vi "PIV_Stats.vi"() -> ()   [LabVIEW 2011]
uses:
  C:/Enflo_Software_SVN/EnFloSW/Anemometry/Anemometry Sub Vis/Controls/PIV_Spot_Data.ctl
  C:/Enflo_Software_SVN/EnFloSW/Anemometry/Anemometry Sub Vis/Controls/PIV_Spot_Cluster.ctl
  <vilib>/Utility/error.llb/DialogType.ctl
  <vilib>/Analysis/1siggen.llb/Ramp Pattern by Samples.vi
  <vilib>/Analysis/NI_AALBase.lvlib
panel:
  out "x+y":dbl[](array[numeric])
  out "size(s)":i32[](array[numeric])
  out "Position Array":dbl[][](array[numeric])
  out "Data Array":dbl[][][](array[numeric])
  out "Variable Loop":i32
  out "Collect data":i32=9857
  in  "Row number":i32=1
  out "Time Loop":i32
  out "Tmax":dbl=0.41379310344827586
  out "# bad vectors":i32[](array[numeric])
  out "# good vectors":i32[](array[numeric])
  out "Max Record Length":i32=3
  out "Numeric Control":i32=2
  out "Variable Names":string[](array[string])=["Record_Length", "CHC", "u_ms", "v_ms", "time_s", "Vel_mag_ms", "Turb_Stats_U_ms", "Turb_Stats_u2_m2s2", "Turb_Stats_u3_m3s3", "Turb_Stats_u4_m4s4", "Turb_Stats_TurbU_%", "Turb_Stats_Skew_u", "Turb_Stats_Kurt_u", "Turb_Stats_V_ms", "Turb_Stats_v2_m2s2", "Turb_Stats_v3_m3s3", "Turb_Stats_v4_m4s4", "Turb_Stats_TurbV_%", "Turb_Stats_Skew_v", "Turb_Stats_Kurt_v", "Turb_Stats_u2v2_m4s4", "Turb_Stats_uv3_m4s4", "Turb_Stats_u3v_m4s4", "Turb_Stats_uv2_m3s3", "Turb_Stats_u2v_m3s3", "Turb_Stats_uv_cc", "Turb_Stats_uv", "Turb_Stats_TKE_J", "Turb_Stats_Error_U_ms", "Turb_Stats_Error_u2_m2s2", "Turb_Stats_Error_u3_m3s3", "Turb_Stats_Error_u4_m4s4", "Turb_Stats_Error_TurbU_%", "Turb_Stats_Error_Skew_u", "Turb_Stats_Error_Kurt_u", "Turb_Stats_Error_V_ms", "Turb_Stats_Error_v2_m2s2", "Turb_Stats_Error_v3_m3s3", "Turb_Stats_Error_v4_m4s4", "Turb_Stats_Error_TurbV_%", "Turb_Stats_Error_Skew_v", "Turb_Stats_Error_Kurt_v", "Turb_Stats_Error_u2v2_m4s4", "Turb_Stats_Error_uv3_m4s4", "Turb_Stats_Error_u3v_m4s4", "Turb_Stats_Error_uv2_m3s3", "Turb_Stats_Error_u2v_m3s3", "Turb_Stats_Error_uv_cc", "Turb_Stats_Error_uv", "Turb_Stats_Error_TKE_J"]
  out "File Paths":path[][](array[path])=[[path "C:/Users/Nick/Desktop/Test/Testing/ENSI_0000.case", path "C:/Users/Nick/Desktop/Test/Testing/ENSI_0000.geo", path "C:/Users/Nick/Desktop/Test/Testing/ENSI_0000.var1", path "C:/Users/Nick/Desktop/Test/Testing/ENSI_0000.var2", path "C:/Users/Nick/Desktop/Test/Testing/ENSI_0000.var3", path "C:/Users/Nick/Desktop/Test/Testing/ENSI_0000.var4", path "C:/Users/Nick/Desktop/Test/Testing/ENSI_0000.var5", path "C:/Users/Nick/Desktop/Test/Testing/ENSI_0000.var6", path "C:/Users/Nick/Desktop/Test/Testing/ENSI_0000.var7", path "C:/Users/Nick/Desktop/Test/Testing/ENSI_0000.var8", path "C:/Users/Nick/Desktop/Test/Testing/ENSI_0000.var9", path "C:/Users/Nick/Desktop/Test/Testing/ENSI_0000.var10", path "C:/Users/Nick/Desktop/Test/Testing/ENSI_0000.var11", path "C:/Users/Nick/Desktop/Test/Testing/ENSI_0000.var12", path "C:/Users/Nick/Desktop/Test/Testing/ENSI_0000.var13", path "C:/Users/Nick/Desktop/Test/Testing/ENSI_0000.var14", path "C:/Users/Nick/Desktop/Test/Testing/ENSI_0000.var15", path "C:/Users/Nick/Desktop/Test/Testing/ENSI_0000.var16", path "C:/Users/Nick/Desktop/Test/Testing/ENSI_0000.var17", path "C:/Users/Nick/Desktop/Test/Testing/ENSI_0000.var18", path "C:/Users/Nick/Desktop/Test/Testing/ENSI_0000.var19", path "C:/Users/Nick/Desktop/Test/Testing/ENSI_0000.var20", path "C:/Users/Nick/Desktop/Test/Testing/ENSI_0000.var21", path "C:/Users/Nick/Desktop/Test/Testing/ENSI_0000.var22", path "C:/Users/Nick/Desktop/Test/Testing/ENSI_0000.var23", path "C:/Users/Nick/Desktop/Test/Testing/ENSI_0000.var24", path "C:/Users/Nick/Desktop/Test/Testing/ENSI_0000.var25", path "C:/Users/Nick/Desktop/Test/Testing/ENSI_0000.var26", path "C:/Users/Nick/Desktop/Test/Testing/ENSI_0000.var27", path "C:/Users/Nick/Desktop/Test/Testing/ENSI_0000.var28", path "C:/Users/Nick/Desktop/Test/Testing/ENSI_0000.var29", path "C:/Users/Nick/Desktop/Test/Testing/ENSI_0000.var30", path "C:/Users/Nick/Desktop/Test/Testing/ENSI_0000.var31", path "C:/Users/Nick/Desktop/Test/Testing/ENSI_0000.var32", path "C:/Users/Nick/Desktop/Test/Testing/ENSI_0000.var33", path "C:/Users/Nick/Desktop/Test/Testing/ENSI_0000.var34", path "C:/Users/Nick/Desktop/Test/Testing/ENSI_0000.var35", path "C:/Users/Nick/Desktop/Test/Testing/ENSI_0000.var36", path "C:/Users/Nick/Desktop/Test/Testing/ENSI_0000.var37", path "C:/Users/Nick/Desktop/Test/Testing/ENSI_0000.var38", path "C:/Users/Nick/Desktop/Test/Testing/ENSI_0000.var39", path "C:/Users/Nick/Desktop/Test/Testing/ENSI_0000.var40", path "C:/Users/Nick/Desktop/Test/Testing/ENSI_0000.var41", path "C:/Users/Nick/Desktop/Test/Testing/ENSI_0000.var42", path "C:/Users/Nick/Desktop/Test/Testing/ENSI_0000.var43", path "C:/Users/Nick/Desktop/Test/Testing/ENSI_0000.var44", path "C:/Users/Nick/Desktop/Test/Testing/ENSI_0000.var45", path "C:/Users/Nick/Desktop/Test/Testing/ENSI_0000.var46", path "C:/Users/Nick/Desktop/Test/Testing/ENSI_0000.var47", path "C:/Users/Nick/Desktop/Test/Testing/ENSI_0000.var48", path "C:/Users/Nick/Desktop/Test/Testing/ENSI_0000.var49", path "C:/Users/Nick/Desktop/Test/Testing/ENSI_0000.var50"], [path "C:/Users/Nick/Desktop/Test/Testing/ENSI_0001.case", path "C:/Users/Nick/Desktop/Test/Testing/ENSI_0001.geo", path "C:/Users/Nick/Desktop/Test/Testing/ENSI_0001.var1", path "C:/Users/Nick/Desktop/Test/Testing/ENSI_0001.var2", path "C:/Users/Nick/Desktop/Test/Testing/ENSI_0001.var3", path "C:/Users/Nick/Desktop/Test/Testing/ENSI_0001.var4", path "C:/Users/Nick/Desktop/Test/Testing/ENSI_0001.var5", path "C:/Users/Nick/Desktop/Test/Testing/ENSI_0001.var6", path "C:/Users/Nick/Desktop/Test/Testing/ENSI_0001.var7", path "C:/Users/Nick/Desktop/Test/Testing/ENSI_0001.var8", path "C:/Users/Nick/Desktop/Test/Testing/ENSI_0001.var9", path "C:/Users/Nick/Desktop/Test/Testing/ENSI_0001.var10", path "C:/Users/Nick/Desktop/Test/Testing/ENSI_0001.var11", path "C:/Users/Nick/Desktop/Test/Testing/ENSI_0001.var12", path "C:/Users/Nick/Desktop/Test/Testing/ENSI_0001.var13", path "C:/Users/Nick/Desktop/Test/Testing/ENSI_0001.var14", path "C:/Users/Nick/Desktop/Test/Testing/ENSI_0001.var15", path "C:/Users/Nick/Desktop/Test/Testing/ENSI_0001.var16", path "C:/Users/Nick/Desktop/Test/Testing/ENSI_0001.var17", path "C:/Users/Nick/Desktop/Test/Testing/ENSI_0001.var18", path "C:/Users/Nick/Desktop/Test/Testing/ENSI_0001.var19", path "C:/Users/Nick/Desktop/Test/Testing/ENSI_0001.var20", path "C:/Users/Nick/Desktop/Test/Testing/ENSI_0001.var21", path "C:/Users/Nick/Desktop/Test/Testing/ENSI_0001.var22", path "C:/Users/Nick/Desktop/Test/Testing/ENSI_0001.var23", path "C:/Users/Nick/Desktop/Test/Testing/ENSI_0001.var24", path "C:/Users/Nick/Desktop/Test/Testing/ENSI_0001.var25", path "C:/Users/Nick/Desktop/Test/Testing/ENSI_0001.var26", path "C:/Users/Nick/Desktop/Test/Testing/ENSI_0001.var27", path "C:/Users/Nick/Desktop/Test/Testing/ENSI_0001.var28", path "C:/Users/Nick/Desktop/Test/Testing/ENSI_0001.var29", path "C:/Users/Nick/Desktop/Test/Testing/ENSI_0001.var30", path "C:/Users/Nick/Desktop/Test/Testing/ENSI_0001.var31", path "C:/Users/Nick/Desktop/Test/Testing/ENSI_0001.var32", path "C:/Users/Nick/Desktop/Test/Testing/ENSI_0001.var33", path "C:/Users/Nick/Desktop/Test/Testing/ENSI_0001.var34", path "C:/Users/Nick/Desktop/Test/Testing/ENSI_0001.var35", path "C:/Users/Nick/Desktop/Test/Testing/ENSI_0001.var36", path "C:/Users/Nick/Desktop/Test/Testing/ENSI_0001.var37", path "C:/Users/Nick/Desktop/Test/Testing/ENSI_0001.var38", path "C:/Users/Nick/Desktop/Test/Testing/ENSI_0001.var39", path "C:/Users/Nick/Desktop/Test/Testing/ENSI_0001.var40", path "C:/Users/Nick/Desktop/Test/Testing/ENSI_0001.var41", path "C:/Users/Nick/Desktop/Test/Testing/ENSI_0001.var42", path "C:/Users/Nick/Desktop/Test/Testing/ENSI_0001.var43", path "C:/Users/Nick/Desktop/Test/Testing/ENSI_0001.var44", path "C:/Users/Nick/Desktop/Test/Testing/ENSI_0001.var45", path "C:/Users/Nick/Desktop/Test/Testing/ENSI_0001.var46", path "C:/Users/Nick/Desktop/Test/Testing/ENSI_0001.var47", path "C:/Users/Nick/Desktop/Test/Testing/ENSI_0001.var48", path "C:/Users/Nick/Desktop/Test/Testing/ENSI_0001.var49", path "C:/Users/Nick/Desktop/Test/Testing/ENSI_0001.var50"], [path "C:/Users/Nick/Desktop/Test/Testing/ENSI_0002.case", path "C:/Users/Nick/Desktop/Test/Testing/ENSI_0002.geo", path "C:/Users/Nick/Desktop/Test/Testing/ENSI_0002.var1", path "C:/Users/Nick/Desktop/Test/Testing/ENSI_0002.var2", path "C:/Users/Nick/Desktop/Test/Testing/ENSI_0002.var3", path "C:/Users/Nick/Desktop/Test/Testing/ENSI_0002.var4", path "C:/Users/Nick/Desktop/Test/Testing/ENSI_0002.var5", path "C:/Users/Nick/Desktop/Test/Testing/ENSI_0002.var6", path "C:/Users/Nick/Desktop/Test/Testing/ENSI_0002.var7", path "C:/Users/Nick/Desktop/Test/Testing/ENSI_0002.var8", path "C:/Users/Nick/Desktop/Test/Testing/ENSI_0002.var9", path "C:/Users/Nick/Desktop/Test/Testing/ENSI_0002.var10", path "C:/Users/Nick/Desktop/Test/Testing/ENSI_0002.var11", path "C:/Users/Nick/Desktop/Test/Testing/ENSI_0002.var12", path "C:/Users/Nick/Desktop/Test/Testing/ENSI_0002.var13", path "C:/Users/Nick/Desktop/Test/Testing/ENSI_0002.var14", path "C:/Users/Nick/Desktop/Test/Testing/ENSI_0002.var15", path "C:/Users/Nick/Desktop/Test/Testing/ENSI_0002.var16", path "C:/Users/Nick/Desktop/Test/Testing/ENSI_0002.var17", path "C:/Users/Nick/Desktop/Test/Testing/ENSI_0002.var18", path "C:/Users/Nick/Desktop/Test/Testing/ENSI_0002.var19", path "C:/Users/Nick/Desktop/Test/Testing/ENSI_0002.var20", path "C:/Users/Nick/Desktop/Test/Testing/ENSI_0002.var21", path "C:/Users/Nick/Desktop/Test/Testing/ENSI_0002.var22", path "C:/Users/Nick/Desktop/Test/Testing/ENSI_0002.var23", path "C:/Users/Nick/Desktop/Test/Testing/ENSI_0002.var24", path "C:/Users/Nick/Desktop/Test/Testing/ENSI_0002.var25", path "C:/Users/Nick/Desktop/Test/Testing/ENSI_0002.var26", path "C:/Users/Nick/Desktop/Test/Testing/ENSI_0002.var27", path "C:/Users/Nick/Desktop/Test/Testing/ENSI_0002.var28", path "C:/Users/Nick/Desktop/Test/Testing/ENSI_0002.var29", path "C:/Users/Nick/Desktop/Test/Testing/ENSI_0002.var30", path "C:/Users/Nick/Desktop/Test/Testing/ENSI_0002.var31", path "C:/Users/Nick/Desktop/Test/Testing/ENSI_0002.var32", path "C:/Users/Nick/Desktop/Test/Testing/ENSI_0002.var33", path "C:/Users/Nick/Desktop/Test/Testing/ENSI_0002.var34", path "C:/Users/Nick/Desktop/Test/Testing/ENSI_0002.var35", path "C:/Users/Nick/Desktop/Test/Testing/ENSI_0002.var36", path "C:/Users/Nick/Desktop/Test/Testing/ENSI_0002.var37", path "C:/Users/Nick/Desktop/Test/Testing/ENSI_0002.var38", path "C:/Users/Nick/Desktop/Test/Testing/ENSI_0002.var39", path "C:/Users/Nick/Desktop/Test/Testing/ENSI_0002.var40", path "C:/Users/Nick/Desktop/Test/Testing/ENSI_0002.var41", path "C:/Users/Nick/Desktop/Test/Testing/ENSI_0002.var42", path "C:/Users/Nick/Desktop/Test/Testing/ENSI_0002.var43", path "C:/Users/Nick/Desktop/Test/Testing/ENSI_0002.var44", path "C:/Users/Nick/Desktop/Test/Testing/ENSI_0002.var45", path "C:/Users/Nick/Desktop/Test/Testing/ENSI_0002.var46", path "C:/Users/Nick/Desktop/Test/Testing/ENSI_0002.var47", path "C:/Users/Nick/Desktop/Test/Testing/ENSI_0002.var48", path "C:/Users/Nick/Desktop/Test/Testing/ENSI_0002.var49", path "C:/Users/Nick/Desktop/Test/Testing/ENSI_0002.var50"]]
  out "ALL filepath":path=path "C:/Users/Nick/Desktop/Test/Testing/ENSI_all.case"
  in  "Invert V":bool
  in  "Invert U":bool
  in  "XYZ Translation":dbl[](array[numeric])=[0.0, 0.0, 0.0]
  in  "PIV Meas Plane":enum16{"XY", "YZ", "XZ"}(ring)=enum."XZ"
  out "time s":dbl[](array[numeric])=[0.0, 0.20689655172413793, 0.41379310344827586]
  in  "PIV Freq (Hz)":dbl=7.25
  out "File Array":path[](array[path])=[path "T:/Ensight_Data/NACA0015/NACA0015_NM_A/Test_A_Trans/New folder/Test_A000000.T076.D000.P000.H000.L.vec", path "T:/Ensight_Data/NACA0015/NACA0015_NM_A/Test_A_Trans/New folder/Test_A000001.T076.D000.P000.H000.L.vec", path "T:/Ensight_Data/NACA0015/NACA0015_NM_A/Test_A_Trans/New folder/Test_A000002.T076.D000.P000.H000.L.vec"]
  out "# total vectors":i32=9858
  in  "Case Name":string="Testing"
  in  "Data Folder":path=path "T:/Ensight_Data/NACA0015/NACA0015_NM_A/Test_A_Trans/New folder"
  in  "Output Directory":path=path "C:/Users/Nick/Desktop/Test"
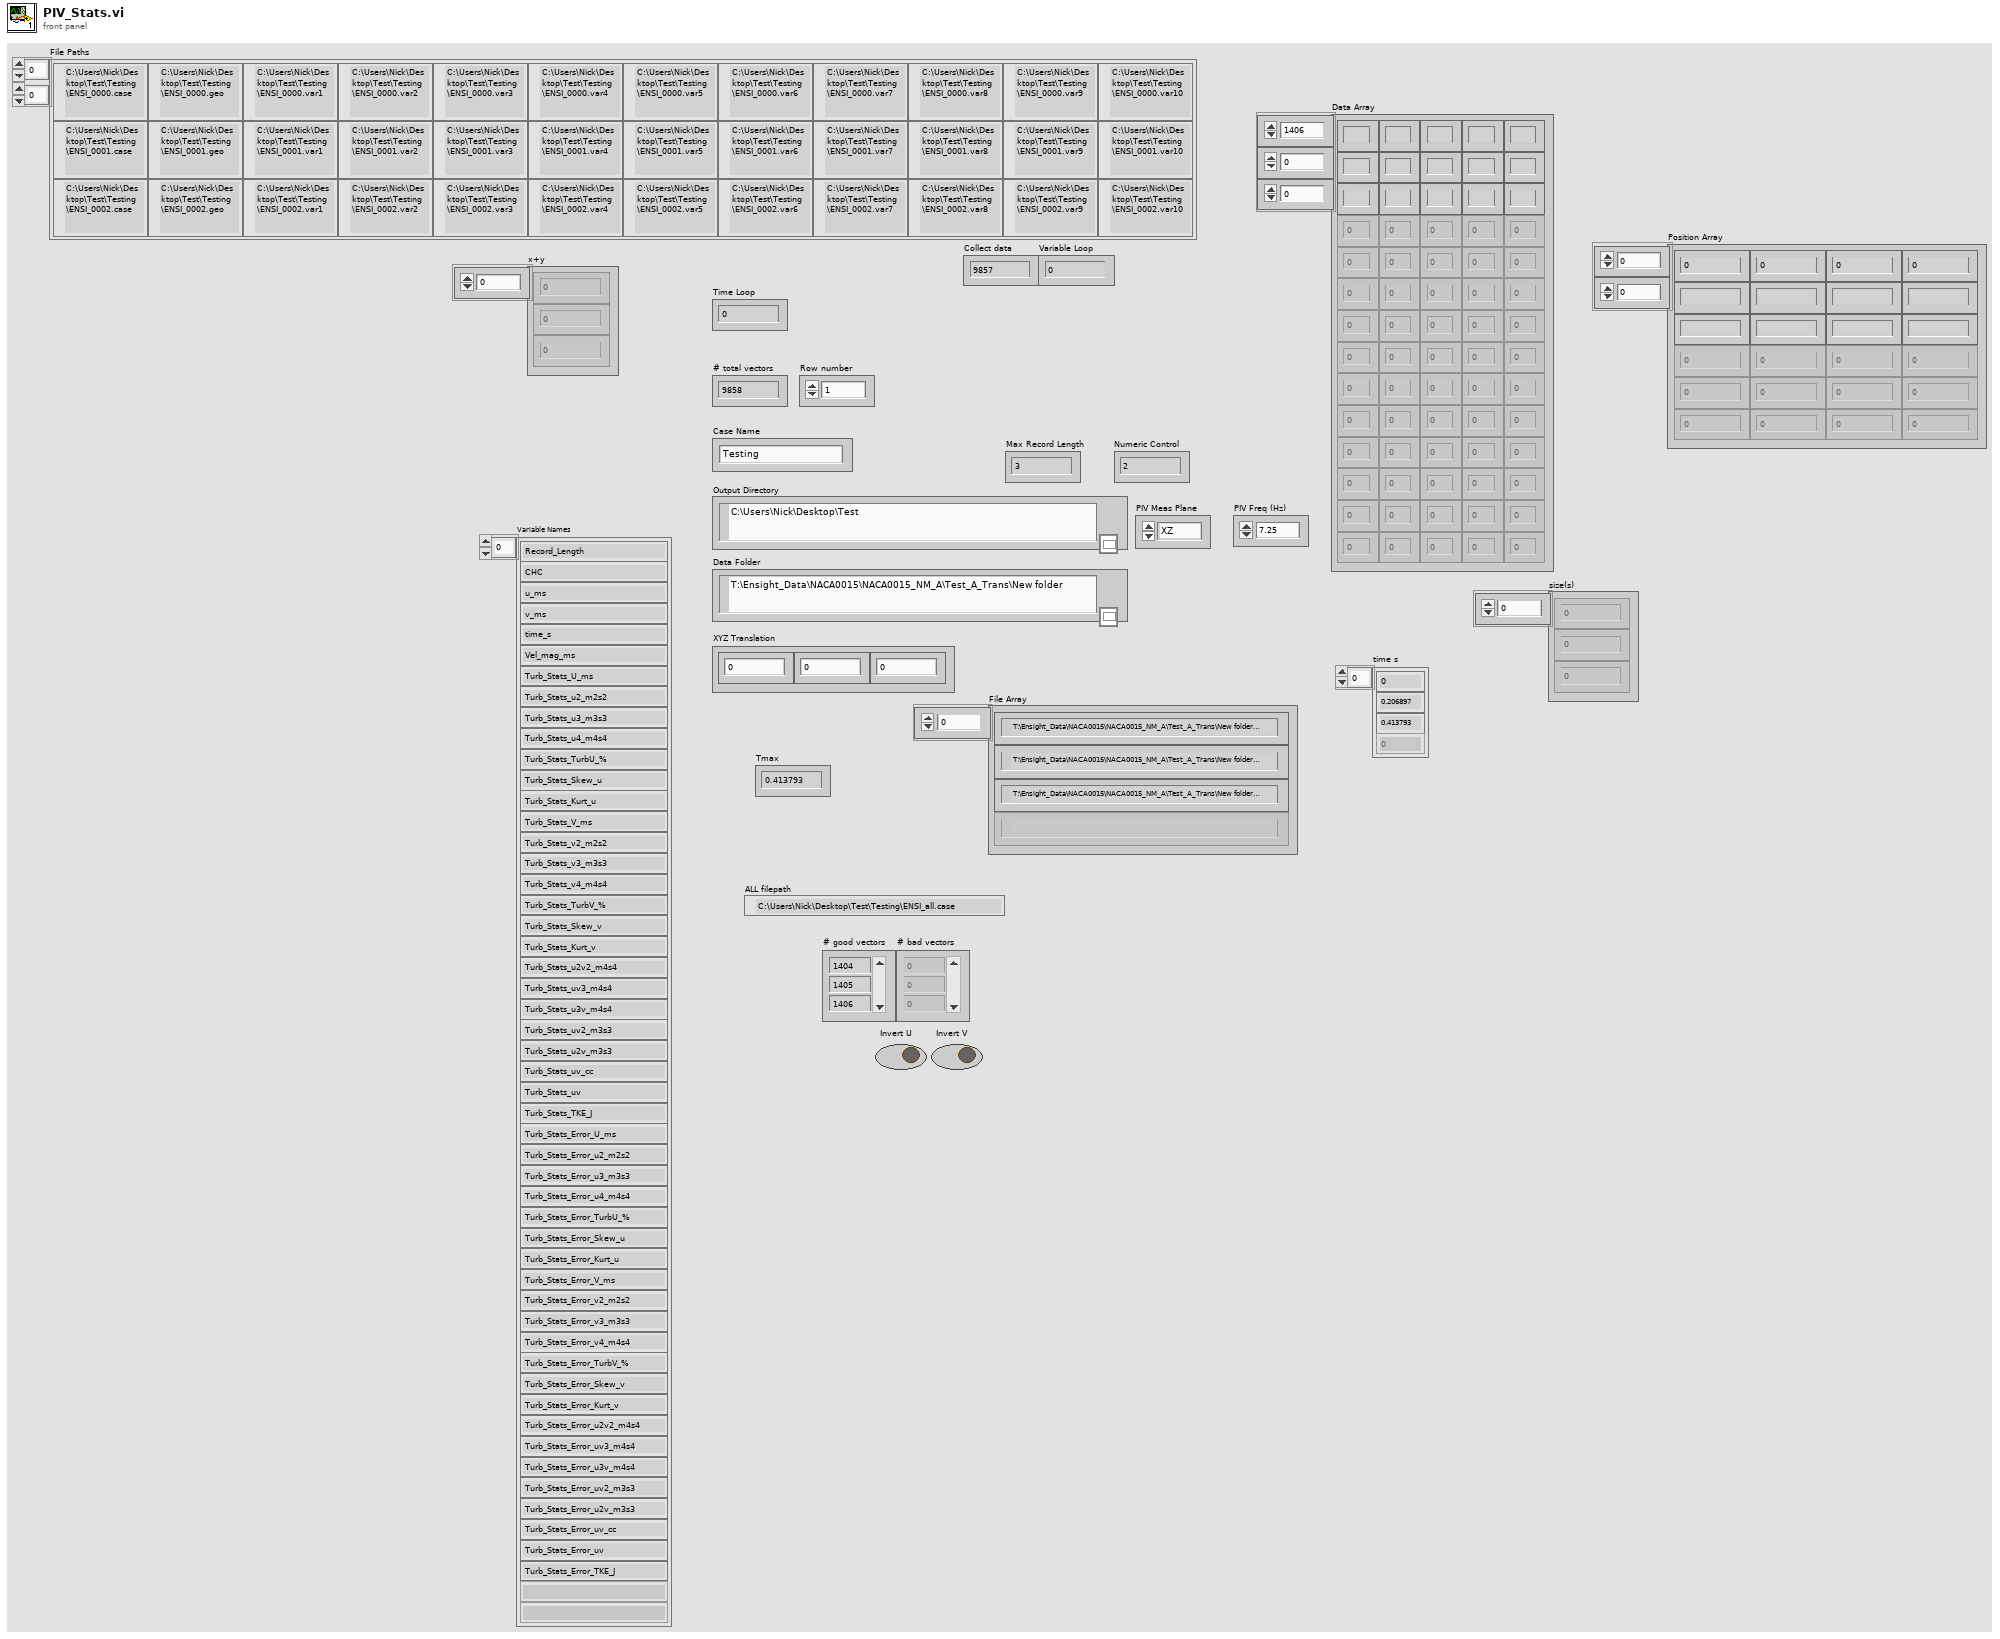
[diagram p1: front panel]
types:
  T1 = typedef "PIV_Spot_Data.ctl" = T2[]
  T2 = typedef "PIV_Spot_Cluster.ctl" = cluster{"Record Length":dbl, "CHC":dbl[], "u m/s":dbl[], "v m/s":dbl[], "time s":dbl[], "Vel mag m/s":dbl[], "XYZ Position":dbl[], " Turb Stats":cluster{"U m/s":dbl, "u2 m2/s2":dbl, "u3 m3/s3":dbl, "u4 m4/s4":dbl, "TurbU %":dbl, "Skew_u":dbl, "Kurt_u":dbl, "V m/s":dbl, "v2 m2/s2":dbl, "v3 m3/s3":dbl, "v4 m4/s4":dbl, "TurbV %":dbl, "Skew_v":dbl, "Kurt_v":dbl, "u2v2 m4/s4":dbl, "uv3 m4/s4":dbl, "u3v m4/s4":dbl, "uv2 m3/s3":dbl, "u2v m3/s3":dbl, "uv_cc":dbl, "uv":dbl, "TKE J":dbl}[], "Turb Stats Error":cluster{"U m/s":dbl, "u2 m2/s2":dbl, "u3 m3/s3":dbl, "u4 m4/s4":dbl, "TurbU %":dbl, "Skew_u":dbl, "Kurt_u":dbl, "V m/s":dbl, "v2 m2/s2":dbl, "v3 m3/s3":dbl, "v4 m4/s4":dbl, "TurbV %":dbl, "Skew_v":dbl, "Kurt_v":dbl, "u2v2 m4/s4":dbl, "uv3 m4/s4":dbl, "u3v m4/s4":dbl, "uv2 m3/s3":dbl, "u2v m3/s3":dbl, "uv_cc":dbl, "uv":dbl, "TKE J":dbl}[]}
  T3 = cluster{"U m/s":dbl, "u2 m2/s2":dbl, "u3 m3/s3":dbl, "u4 m4/s4":dbl, "TurbU %":dbl, "Skew_u":dbl, "Kurt_u":dbl, "V m/s":dbl, "v2 m2/s2":dbl, "v3 m3/s3":dbl, "v4 m4/s4":dbl, "TurbV %":dbl, "Skew_v":dbl, "Kurt_v":dbl, "u2v2 m4/s4":dbl, "uv3 m4/s4":dbl, "u3v m4/s4":dbl, "uv2 m3/s3":dbl, "u2v m3/s3":dbl, "uv_cc":dbl, "uv":dbl, "TKE J":dbl}
  T4 = cluster{"U m/s":dbl, "u2 m2/s2":dbl, "u3 m3/s3":dbl, "u4 m4/s4":dbl, "TurbU %":dbl, "Skew_u":dbl, "Kurt_u":dbl, "V m/s":dbl, "v2 m2/s2":dbl, "v3 m3/s3":dbl, "v4 m4/s4":dbl, "TurbV %":dbl, "Skew_v":dbl, "Kurt_v":dbl, "u2v2 m4/s4":dbl, "uv3 m4/s4":dbl, "u3v m4/s4":dbl, "uv2 m3/s3":dbl, "u2v m3/s3":dbl, "uv_cc":dbl, "uv":dbl, "TKE J":dbl}[]
  T5 = typedef "DialogType.ctl" = u16
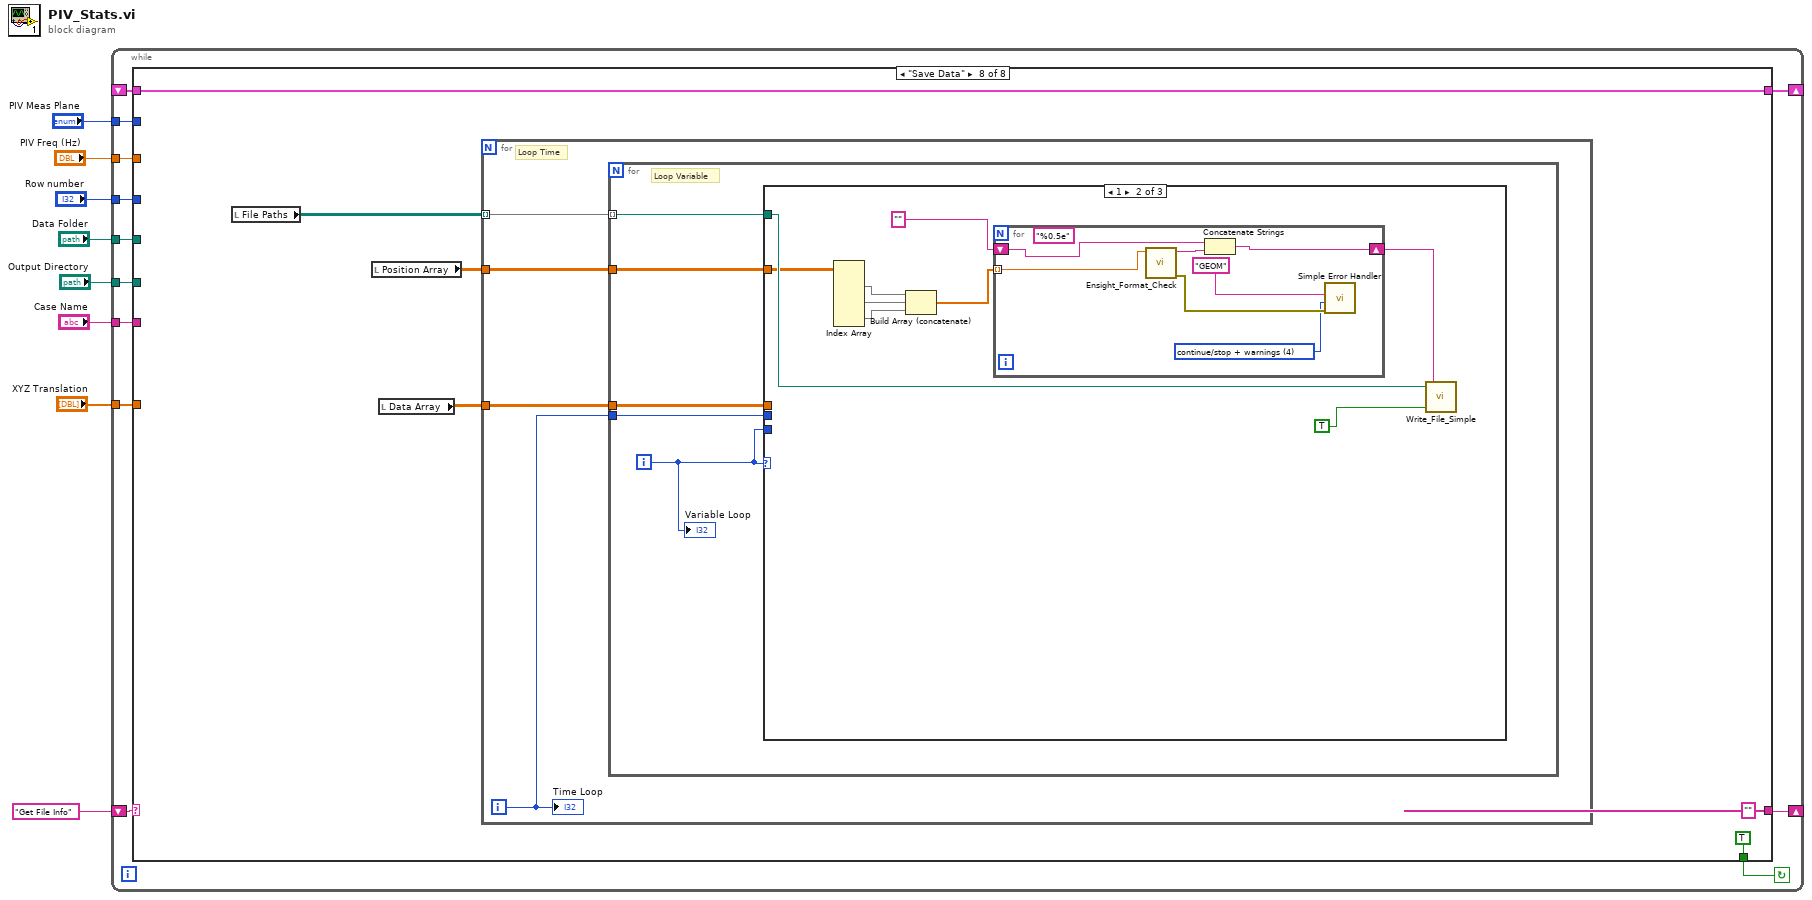
[diagram p0: block diagram]
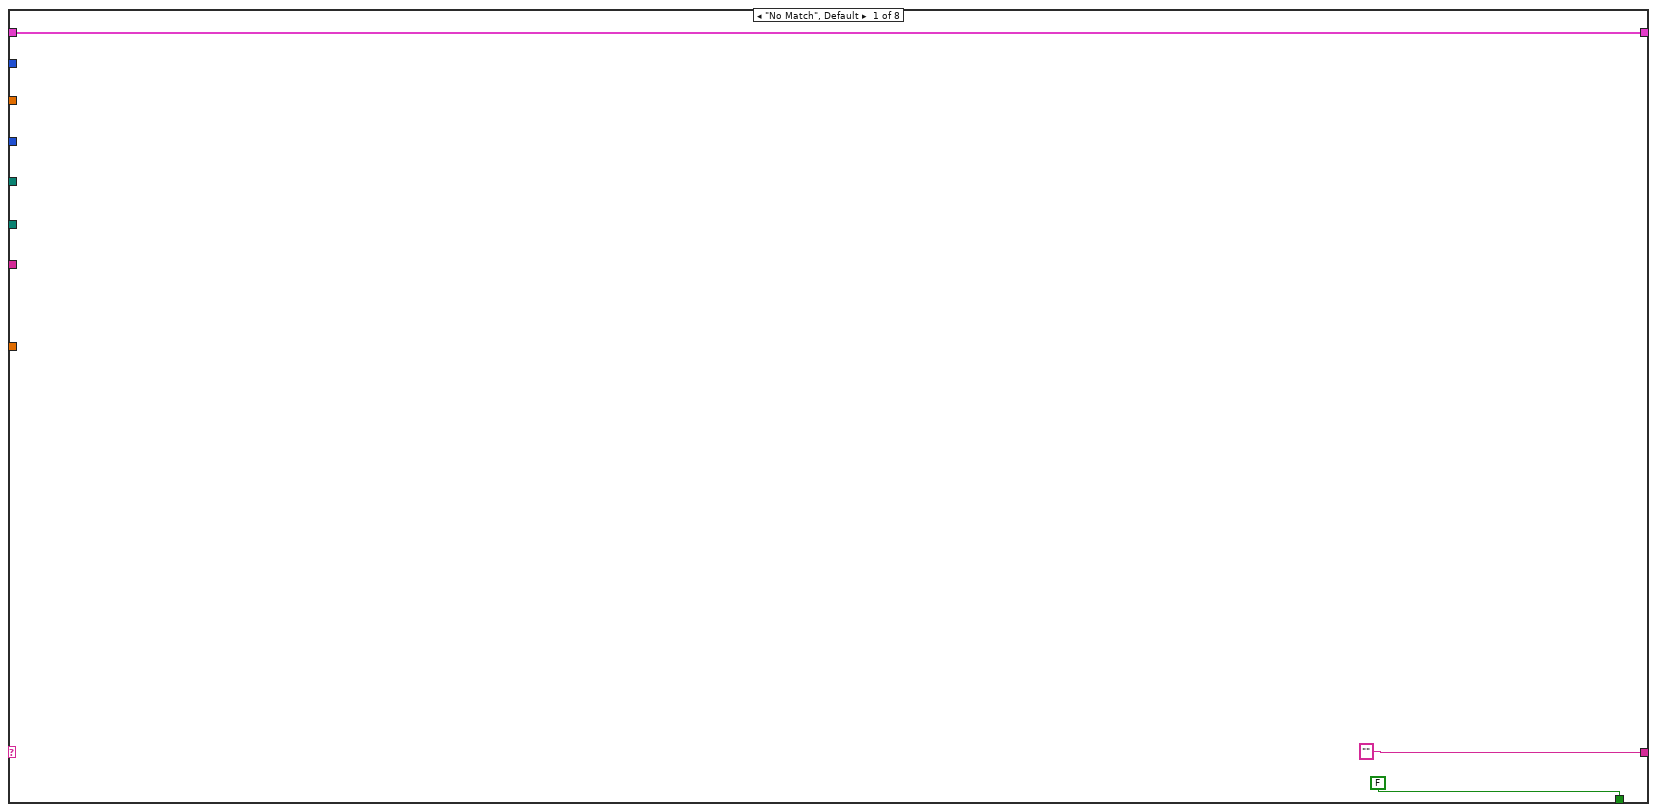
[diagram p2: hidden frame]
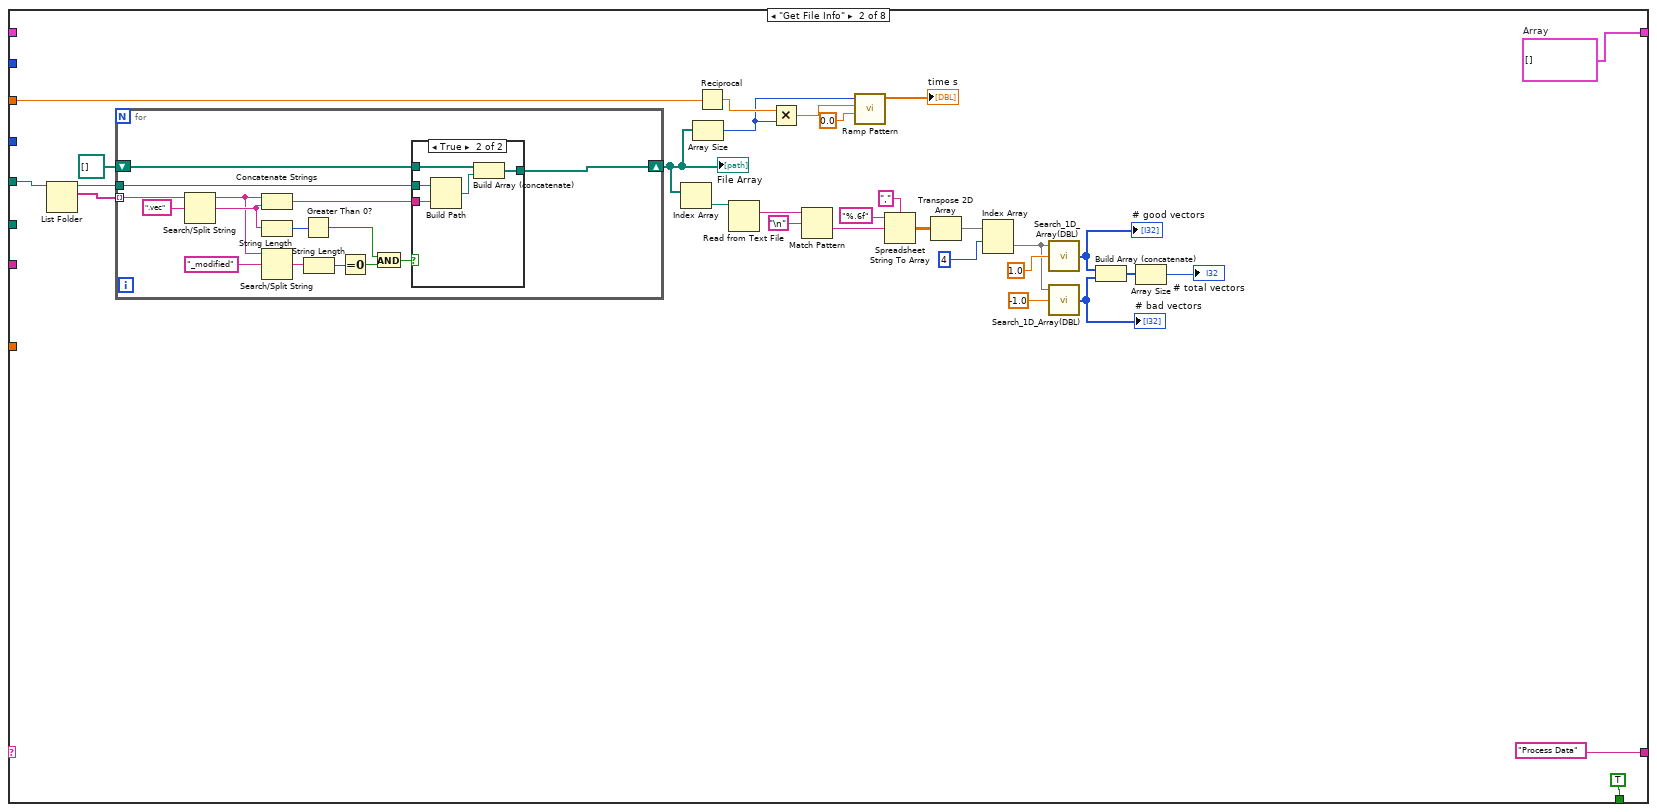
[diagram p3: hidden frame]
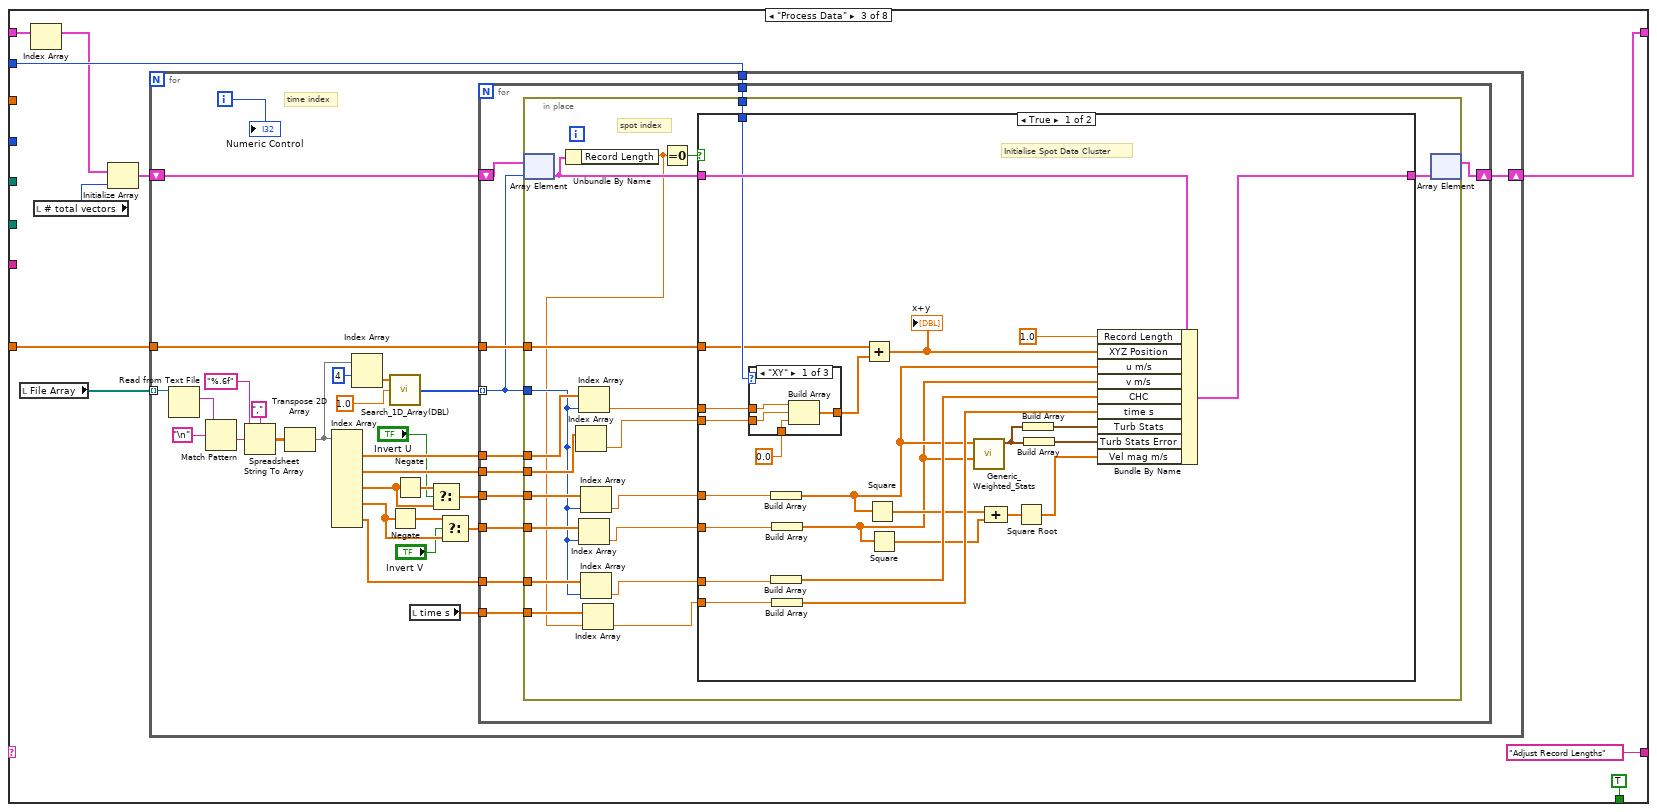
[diagram p5: hidden frame]
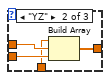
[diagram p6: hidden frame]
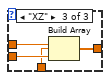
[diagram p7: hidden frame]
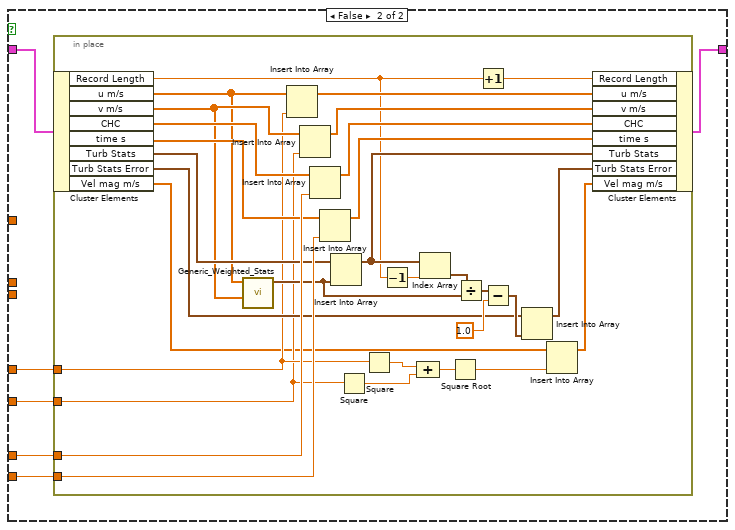
[diagram p8: hidden frame]
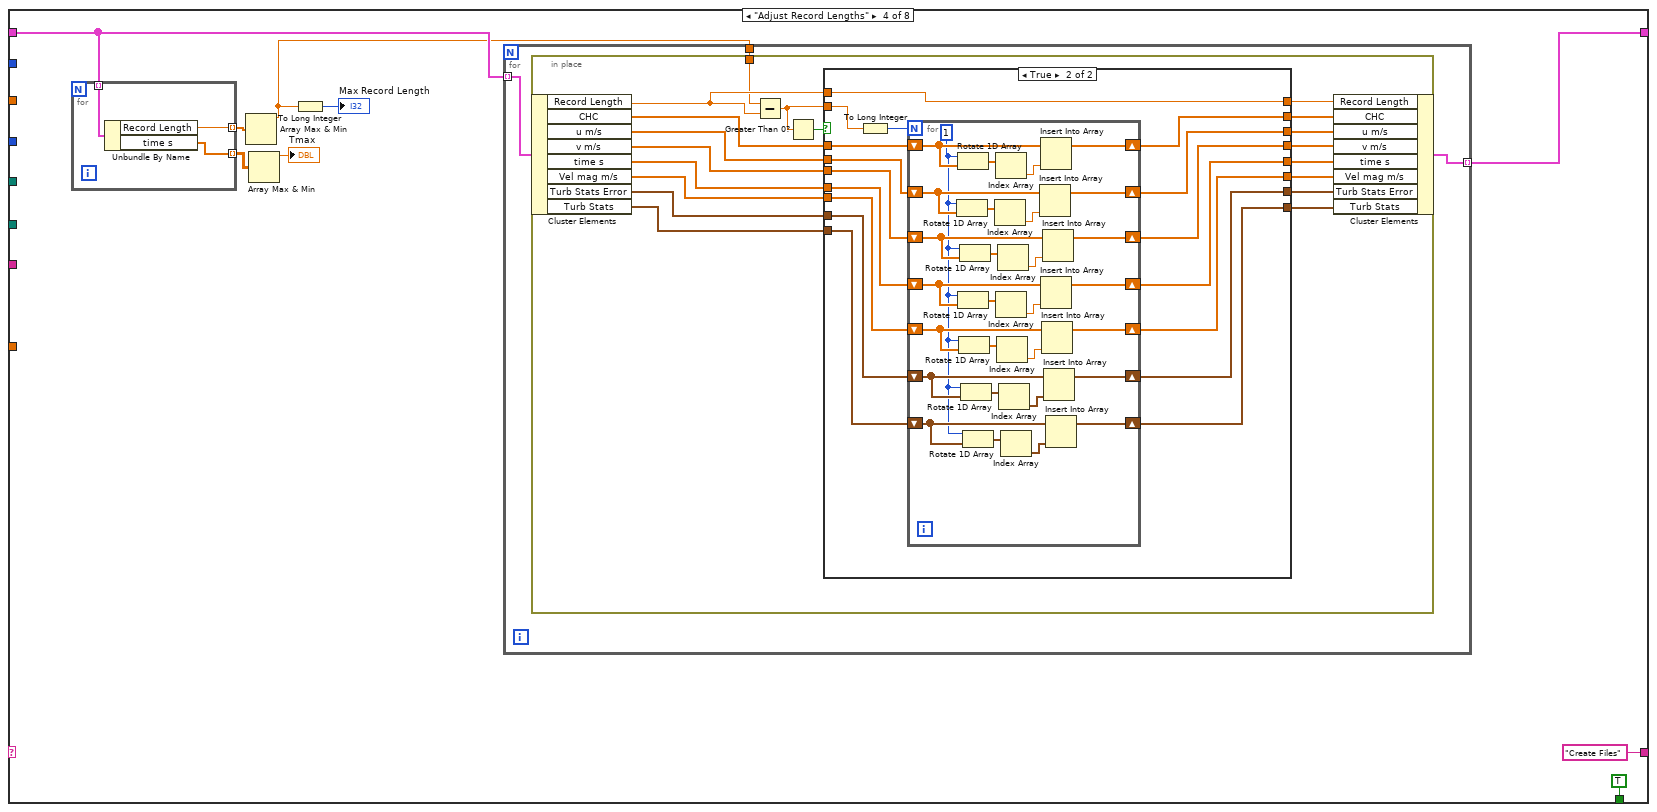
[diagram p9: hidden frame]
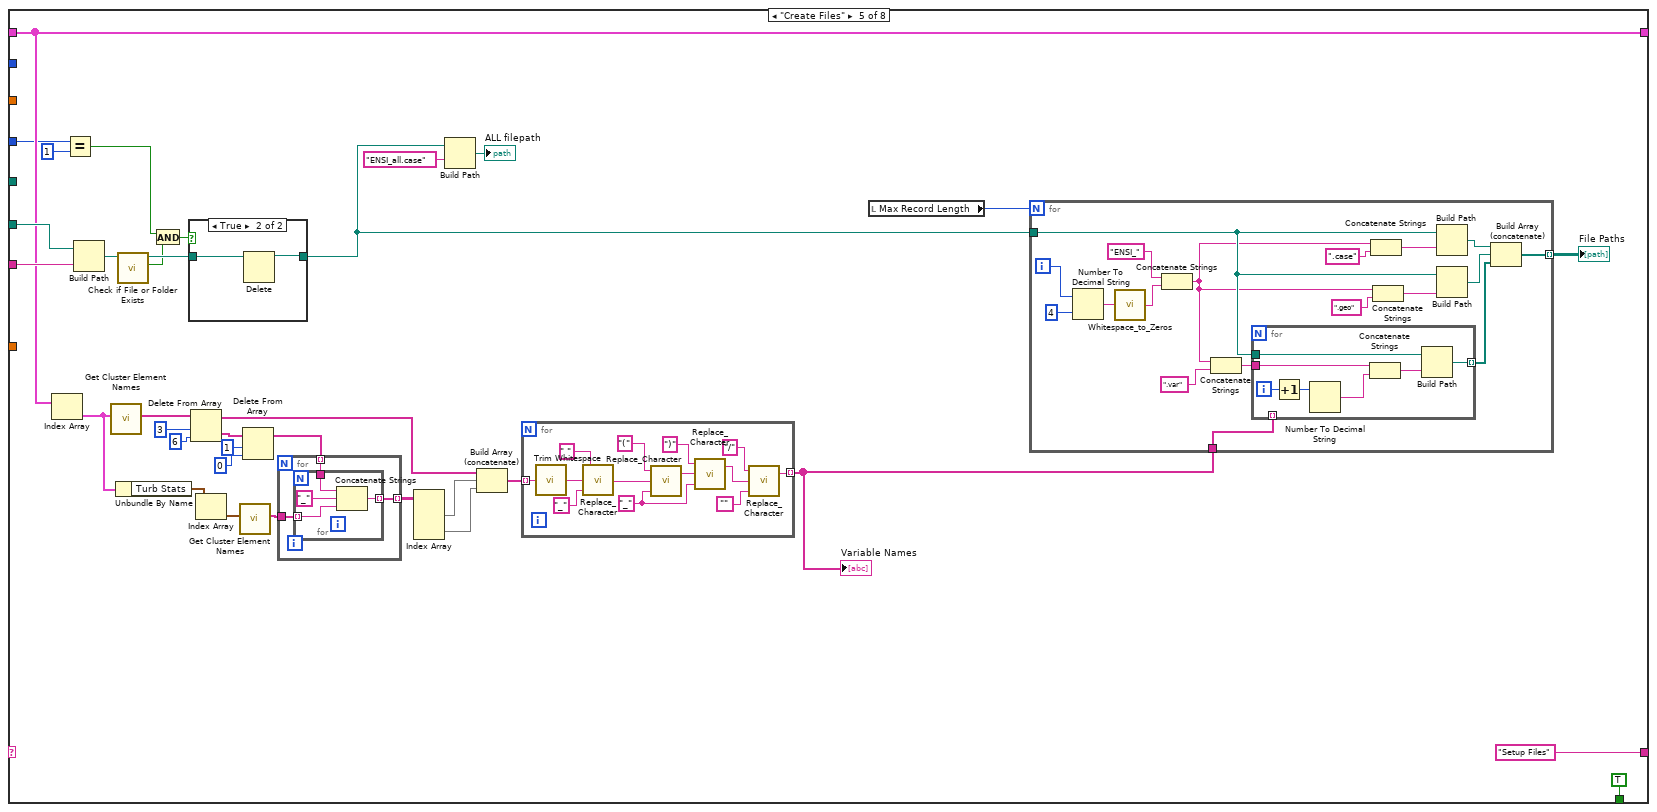
[diagram p11: hidden frame]
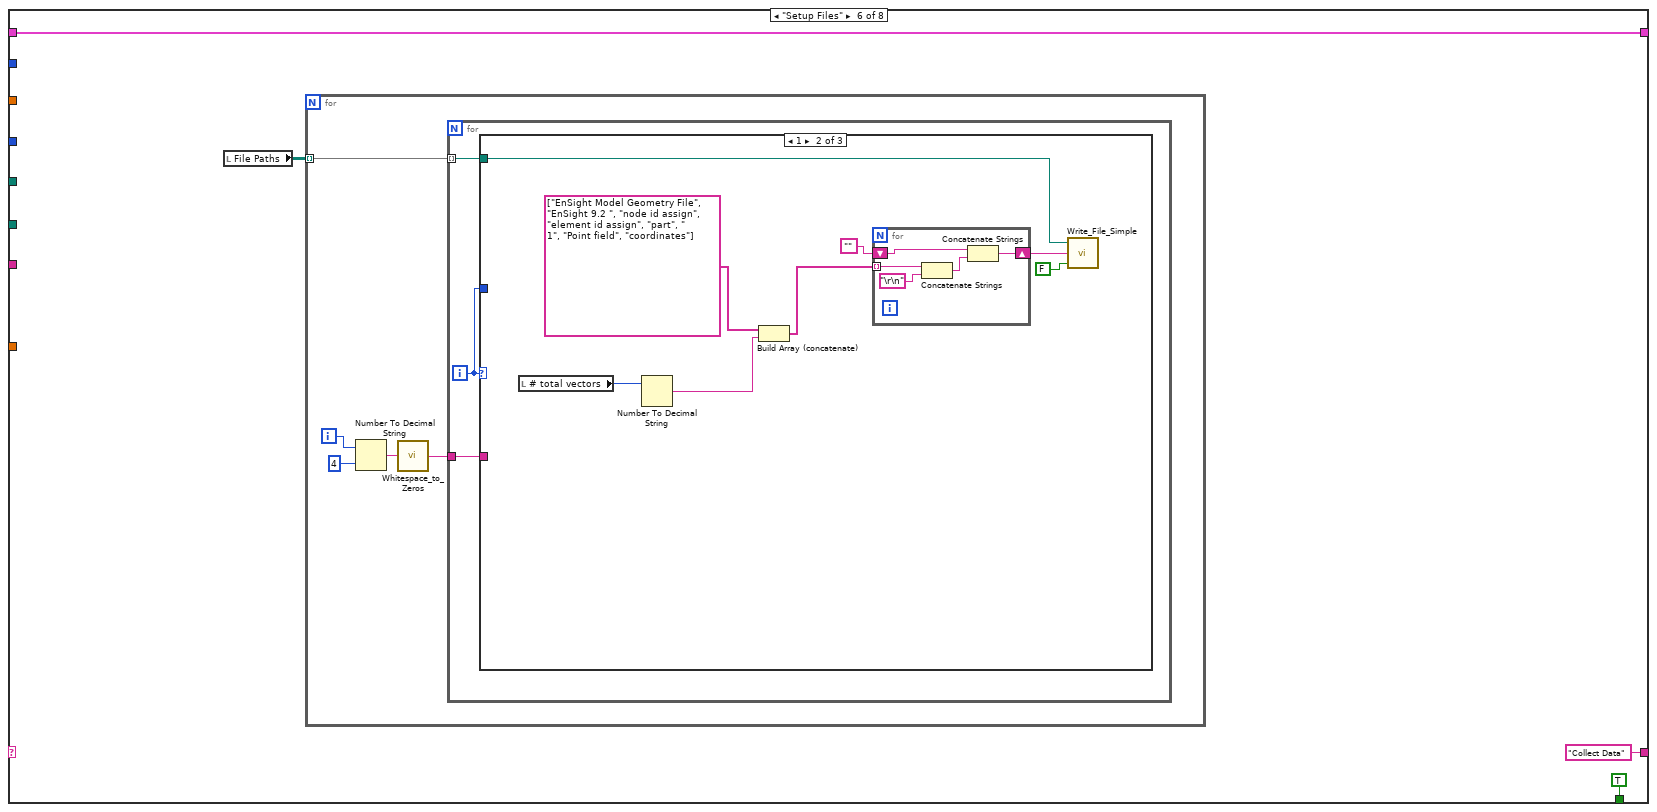
[diagram p13: hidden frame]
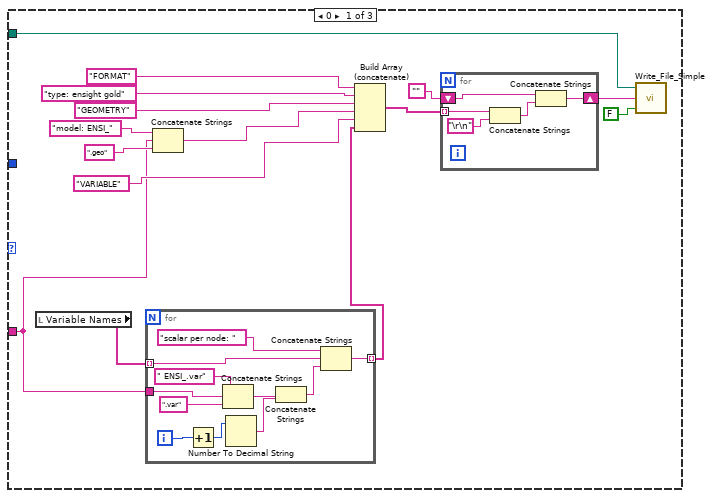
[diagram p14: hidden frame]
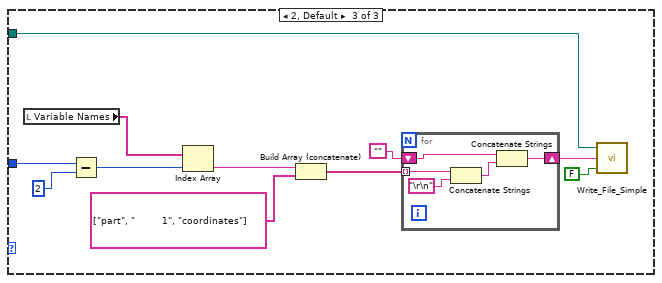
[diagram p15: hidden frame]
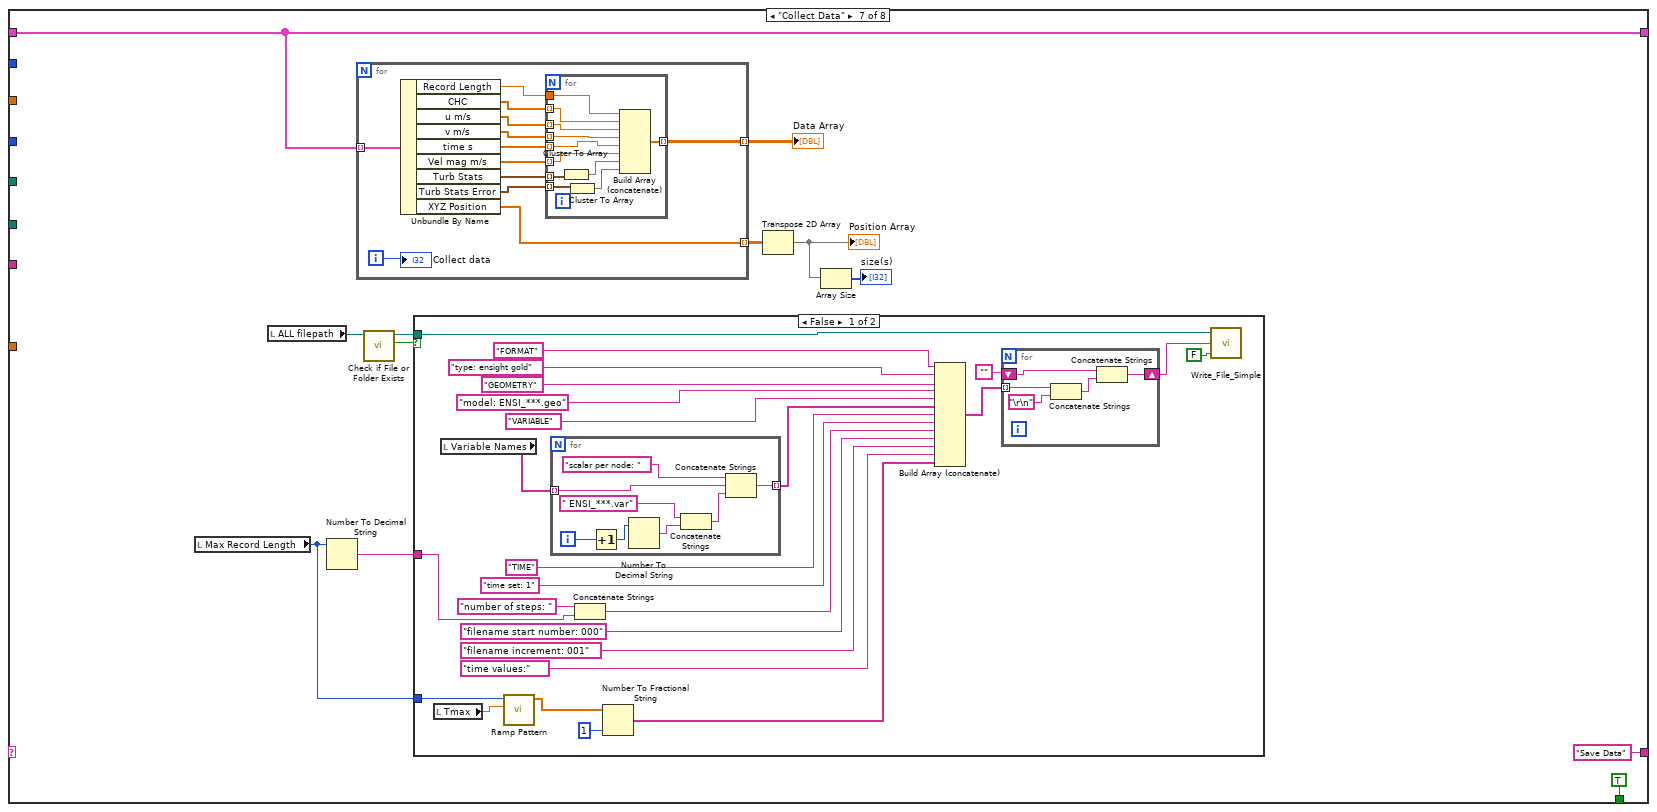
[diagram p16: hidden frame]
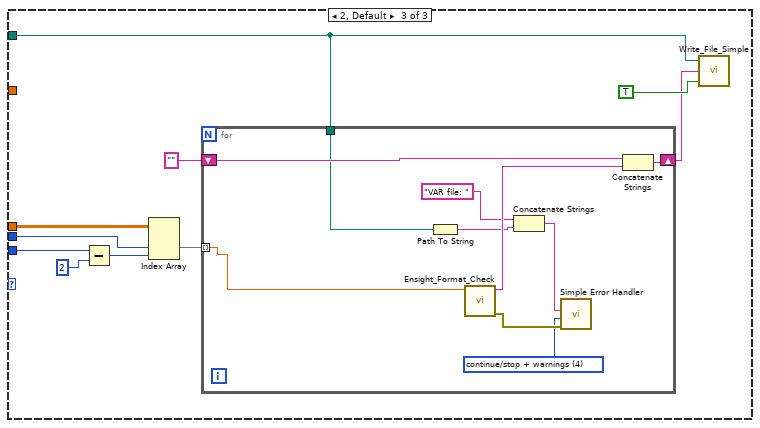
[diagram p19: hidden frame]
diagram:
  n1 = while {
    shift-right: [w19] -> _
    shift-left: "Get File Info" -> [w20]
    tunnel: "Data Folder" -> [w18]
    tunnel: "Output Directory" -> [w16]
    tunnel: "Case Name" -> [w15]
    tunnel: "PIV Freq (Hz)" -> [w14]
    tunnel: "PIV Meas Plane" -> [w13]
    tunnel: "XYZ Translation" -> [w12]
    shift-right: [w11] -> _
    shift-left: _ -> [w10]
    tunnel: "Row number" -> [w9]
    stop <- w17 continue-if-true
    n2 = case shown="\"Save Data\"" w20 {
      tunnel: ["" "Process Data" "Adjust Record Lengths" "Create Files" "Setup Files" ("t") "Collect Data" ("t") "Save Data" ("t") "" ("t")] -> w19
      tunnel: w18 -> [_ w48 _ _ _ _ _ _]
      tunnel: [FALSE TRUE TRUE TRUE TRUE TRUE TRUE TRUE] -> w17
      tunnel: w16 -> [_ _ _ _ w334 _ _ _]
      tunnel: w15 -> [_ _ _ _ w335 _ _ _]
      tunnel: w14 -> [_ w41 _ _ _ _ _ _]
      tunnel: w13 -> [_ _ w80 _ _ _ _ _]
      tunnel: w12 -> [_ _ w79 _ _ _ _ _]
      tunnel: [w21 w25 w77 w223 w318 w387 w463 w535] -> w11
      tunnel: w10 -> [w21 _ w76 w222 w318 w387 w463 w535]
      tunnel: w9 -> [_ _ _ _ w313 _ _ _]
      frame "No Match", Default {
      }
      frame "Get File Info" {
        w25 = T1 []  # Array
        n3 = List Folder(path=w48) -> (path out=w50:path, filenames=w51:string[])  [unwired: 3 in, 2 out]
        n4 = for {
          tunnel: w51 -> [w68] mode=indexing
          shift-right: [w61] -> w33
          shift-left: path[] [] -> [w63]
          tunnel: w50 -> [w62]
          n5 = Search/Split String(string=w68, search string/char (-)=".vec") -> (substring before match=w59:string, match + rest of string=w65:string)  [unwired: 1 in, 1 out]
          n6 = Concatenate Strings(w59, w65) -> (w64:string)
          n7 = String Length(string=w65) -> (length=w66:i32)
          n8 = Search/Split String(string=w59, search string/char (-)="_modified") -> (match + rest of string=w57:string)  [unwired: 1 in, 2 out]
          n9 = Greater Than 0?(x=w66) -> (x > 0?=w60:bool)
          n10 = String Length(string=w57) -> (length=w56:i32)
          n11 = Equal To 0?(x=w56) -> (x = 0?=w55:bool)
          n12 = And(x=w60, y=w55) -> (x .and. y?=w54:bool)
          n13 = case shown="True" w54 {
            tunnel: w64 -> [_ w74]
            tunnel: w63 -> [w69 w70]
            tunnel: w62 -> [_ w73]
            tunnel: [w69 w71] -> w61
            frame False {
            }
            frame True {
              n14 = Build Path(base path=w73, name or relative path=w74) -> (appended path=w72:path)
              n15 = Build Array (concatenate)(w70, w72) -> (w71:path[])
            }
          }
        }
        "File Array" <- w33
        n16 = Index Array(array=w33) -> (element=w42:path)  [unwired: 1 in]
        n17 = Array Size(array=w33) -> (size(s)=w30:i32)
        n18 = Reciprocal(x=w41) -> (1/x=w39:dbl)
        n19 = Read from Text File(file (use dialog)=w42) -> (text=w47:string)  [unwired: 3 in, 3 out]
        n20 = Multiply(x=w39, y=w30) -> (x*y=w40:dbl)
        n21 = Match Pattern(string=w47, regular expression="\n") -> (after substring=w43:string)  [unwired: 1 in, 3 out]
        n22 = call-poly <vilib>:"Ramp Pattern.vi"("start"=0.0, "end"=w40, "samples"=w30) -> ("Ramp Pattern"=→"time s":dbl[])  [unwired: 7 in, 1 out]
        n23 = Spreadsheet String To Array(delimiter (Tab)=",", format string="%.6f", spreadsheet string=w43) -> (array=w34:dbl[][])  [unwired: 1 in]
        n24 = Transpose 2D Array(2D array=w34) -> (transposed array=w36:dbl[][])
        n25 = Index Array(array=w36, index (row)=4) -> (element=w29:dbl[])  [unwired: 1 in]
        n26 = call "Search_1D_Array(DBL).vi"("Array"=w29, "Element Data"=1.0) -> ("Indicies of Elements"=w27:i32[])  [unwired: 7 in]
        "# good vectors" <- w27
        n27 = call "Search_1D_Array(DBL).vi"("Array"=w29, "Element Data"=-1.0) -> ("Indicies of Elements"=w24:i32[])  [unwired: 7 in]
        "# bad vectors" <- w24
        n28 = Build Array (concatenate)(w27, w24) -> (w26:i32[])
        n29 = Array Size(array=w26) -> (size(s)=→"# total vectors":i32)
      }
      frame "Process Data" {
        n30 = local read "File Array"() -> (w81:path[])
        n31 = Index Array(array=w76) -> (element=w75:T2)  [unwired: 1 in]
        n32 = local read "# total vectors"() -> (w78:i32)
        n33 = Initialize Array(w75, w78) -> (w82:T2[])
        n34 = for {
          tunnel: w81 -> [w113] mode=indexing
          shift-right: [w89] -> w77
          shift-left: w82 -> [w106]
          tunnel: w80 -> [w101]
          tunnel: w79 -> [w100]
          i -> [w86]
          # "time index"
          n35 = Read from Text File(file (use dialog)=w113) -> (text=w107:string)  [unwired: 3 in, 3 out]
          n36 = Match Pattern(string=w107, regular expression="\n") -> (after substring=w111:string)  [unwired: 1 in, 3 out]
          n37 = Spreadsheet String To Array(delimiter (Tab)=",", format string="%.6f", spreadsheet string=w111) -> (array=w112:dbl[][])  [unwired: 1 in]
          n38 = Transpose 2D Array(2D array=w112) -> (transposed array=w99:dbl[][])
          n39 = Index Array(array=w99) -> (element #1=w103:dbl[], element #2=w102:dbl[], element #3=w98:dbl[], element #4=w95:dbl[], element #5=w92:dbl[])  [unwired: 10 in]
          n40 = Index Array(array=w99, index (row)=4) -> (element=w88:dbl[])  [unwired: 1 in]
          n41 = call "Search_1D_Array(DBL).vi"("Array"=w88, "Element Data"=1.0) -> ("Indicies of Elements"=w85:i32[])  [unwired: 7 in]
          n42 = Negate(x=w95) -> (-x=w96:dbl[])
          n43 = Negate(x=w98) -> (-x=w97:dbl[])
          n44 = local read "time s"() -> (w104:dbl[])
          n45 = Select(t=w97, s="Invert U", f=w98) -> (s? t:f=w91:dbl[])
          n46 = Select(t=w96, s="Invert V", f=w95) -> (s? t:f=w90:dbl[])
          n47 = for {
            tunnel: w104 -> [w117]
            tunnel: w103 -> [w124]
            tunnel: w102 -> [w123]
            tunnel: w101 -> [w122]
            tunnel: w100 -> [w121]
            tunnel: w92 -> [w118]
            tunnel: w91 -> [w120]
            tunnel: w90 -> [w119]
            tunnel: w85 -> [w114] mode=indexing
            shift-right: [w115] -> w89
            shift-left: w106 -> [w116]
            n48 = in-place {
              in-place-border: w124 -> [w143]
              in-place-border: w123 -> [w142]
              in-place-border: w122 -> [w141]
              in-place-border: w121 -> [w140]
              in-place-border: w120 -> [w139]
              in-place-border: w119 -> [w138]
              in-place-border: w118 -> [w137]
              in-place-border: w117 -> [w136]
              in-place-border: w114 -> [w126]
              # "spot index"
              n49 = in-place-array #1(w116, w114) -> (w128:T2)
              n50 = Unbundle By Name(w128) -> ("Record Length"=w125:dbl)
              n51 = Index Array(array=w142, index=w126) -> (element=w134:dbl)
              n52 = Index Array(array=w143, index=w126) -> (element=w135:dbl)
              n53 = Index Array(array=w138, index=w126) -> (element=w132:dbl)
              n54 = Index Array(array=w139, index=w126) -> (element=w133:dbl)
              n55 = Index Array(array=w137, index=w126) -> (element=w131:dbl)
              n56 = Index Array(array=w136, index=w125) -> (element=w130:dbl)
              n57 = Equal To 0?(x=w125) -> (x = 0?=w129:bool)
              n58 = case shown="True" w129 {
                tunnel: [w167 w186] -> w127
                tunnel: w132 -> [w155 w183]
                tunnel: w128 -> [w168 w185]
                tunnel: w135 -> [w164 _]
                tunnel: w134 -> [w163 _]
                tunnel: w141 -> [w165 _]
                tunnel: w140 -> [w161 _]
                tunnel: w133 -> [w158 w184]
                tunnel: w131 -> [w157 w182]
                tunnel: w130 -> [w154 w181]
                frame True {
                  # "Initialise Spot Data Cluster"
                  n59 = case shown="\"XY\"" w165 {
                    tunnel: w164 -> [w170 w176 w180]
                    tunnel: w163 -> [w171 w175 w179]
                    tunnel: 0.0 ("element") -> [w172 w174 w178]
                    tunnel: [w169 w173 w177] -> w162
                    frame "XY" {
                      n60 = Build Array(w170, w171, w172) -> (w169:dbl[])
                    }
                    frame "YZ" {
                      n61 = Build Array(w174, w176, w175) -> (w173:dbl[])
                    }
                    frame "XZ" {
                      n62 = Build Array(w180, w178, w179) -> (w177:dbl[])
                    }
                  }
                  n63 = Build Array(w158) -> (w149:dbl[])
                  n64 = Build Array(w157) -> (w156:dbl[])
                  n65 = Build Array(w155) -> (w147:dbl[])
                  n66 = Build Array(w154) -> (w153:dbl[])
                  n67 = Add(x=w161, y=w162) -> (x+y=w160:dbl[])
                  "x+y" <- w160
                  n68 = Square(x=w149) -> (x^2=w148:dbl[])
                  n69 = Square(x=w147) -> (x^2=w146:dbl[])
                  n70 = call "Generic_Weighted_Stats.vi"("v"=w147, "u"=w149) -> ("Turbulence Statistics"=w151:T3)  [unwired: 9 in]
                  n71 = Compound Arithmetic op=ADD(w148, w146) -> (w145:dbl[])
                  n72 = Square Root(x=w145) -> (sqrt(x)=w144:dbl[])
                  n73 = Build Array(w151) -> (w152:T4)
                  n74 = Build Array(w151) -> (w150:T4)
                  n75 = Bundle By Name(cluster=w168, "Record Length"=1.0, "XYZ Position"=w160, "u m/s"=w149, "v m/s"=w147, "CHC"=w156, "time s"=w153, "Turb Stats"=w152, "Turb Stats Error"=w150, "Vel mag m/s"=w144) -> (w167:T2)
                }
                frame False {
                  n76 = in-place {
                    in-place-border: w184 -> [w193]
                    in-place-border: w183 -> [w192]
                    in-place-border: w182 -> [w213]
                    in-place-border: w181 -> [w211]
                    n77 = in-place-cluster #2(w185) -> ("Record Length"=w204:dbl, "u m/s"=w206:dbl[], "v m/s"=w207:dbl[], "CHC"=w214:dbl[], "time s"=w208:dbl[], "Turb Stats"=w209:T4, "Turb Stats Error"=w197:T4, "Vel mag m/s"=w190:dbl[])
                    n78 = call "Generic_Weighted_Stats.vi"("v"=w207, "u"=w206) -> ("Turbulence Statistics"=w201:T3)  [unwired: 9 in]
                    n79 = Insert Into Array(array=w206, new element=w193) -> (w216:dbl[])  [unwired: 1 in]
                    n80 = Insert Into Array(array=w207, new element=w192) -> (w215:dbl[])  [unwired: 1 in]
                    n81 = Insert Into Array(array=w214, new element=w213) -> (w212:dbl[])  [unwired: 1 in]
                    n82 = Insert Into Array(array=w208, new element=w211) -> (w210:dbl[])  [unwired: 1 in]
                    n83 = Insert Into Array(array=w209, new element=w201) -> (w205:T4)  [unwired: 1 in]
                    n84 = Square(x=w192) -> (x^2=w195:dbl)
                    n85 = Square(x=w193) -> (x^2=w196:dbl)
                    n86 = Decrement(x=w204) -> (x-1=w203:dbl)
                    n87 = Compound Arithmetic op=ADD(w196, w195) -> (w194:dbl)
                    n88 = Index Array(array=w205, index=w203) -> (element=w202:T3)
                    n89 = Square Root(x=w194) -> (sqrt(x)=w188:dbl)
                    n90 = Divide(x=w202, y=w201) -> (x/y=w200:T3)
                    n91 = Increment(x=w204) -> (x+1=w187:dbl)
                    n92 = Subtract(x=w200, y=1.0 ("Record Length")) -> (x-y=w198:T3)
                    n93 = Insert Into Array(array=w197, new element=w198) -> (w191:T4)  [unwired: 1 in]
                    n94 = Insert Into Array(array=w190, new element=w188) -> (w189:dbl[])  [unwired: 1 in]
                    n95 = in-place-cluster #2("Record Length"=w187, "u m/s"=w216, "v m/s"=w215, "CHC"=w212, "time s"=w210, "Turb Stats"=w205, "Turb Stats Error"=w191, "Vel mag m/s"=w189) -> (w186:T2)
                  }
                }
              }
              n96 = in-place-array #1(w127) -> (w115:T2[])  [unwired: 1 out]
            }
          }
          "Numeric Control" <- w86
        }
      }
      frame "Adjust Record Lengths" {
        n97 = for {
          tunnel: w222 -> [w228] mode=indexing
          tunnel: [w227] -> w221 mode=indexing
          tunnel: [w226] -> w218 mode=indexing
          n98 = Unbundle By Name(w228) -> ("Record Length"=w227:dbl, "time s"=w226:dbl[])
        }
        n99 = Array Max & Min(array=w221) -> (max value=w220:dbl)  [unwired: 3 out]
        n100 = Array Max & Min(array=w218) -> (max value=→"Tmax":dbl)  [unwired: 3 out]
        n101 = To Long Integer(number=w220) -> (32bit integer=→"Max Record Length":i32)
        n102 = for {
          tunnel: w222 -> [w231] mode=indexing
          tunnel: w220 -> [w230]
          tunnel: [w229] -> w223 mode=indexing
          n103 = in-place {
            in-place-border: w230 -> [w232]
            n104 = in-place-cluster #3(w231) -> ("Record Length"=w233:dbl, "CHC"=w246:dbl[], "u m/s"=w244:dbl[], "v m/s"=w242:dbl[], "time s"=w240:dbl[], "Vel mag m/s"=w238:dbl[], "Turb Stats Error"=w236:T4, "Turb Stats"=w234:T4)
            n105 = Subtract(x=w232, y=w233) -> (x-y=w249:dbl)
            n106 = Greater Than 0?(x=w249) -> (x > 0?=w250:bool)
            n107 = case shown="True" w250 {
              tunnel: w249 -> [_ w274]
              tunnel: [w251 w259] -> w248
              tunnel: [w258 w273] -> w247
              tunnel: w246 -> [w258 w275]
              tunnel: [w257 w266] -> w245
              tunnel: w244 -> [w257 w272]
              tunnel: [w256 w265] -> w243
              tunnel: w242 -> [w256 w271]
              tunnel: [w255 w264] -> w241
              tunnel: w240 -> [w255 w270]
              tunnel: [w254 w263] -> w239
              tunnel: w238 -> [w254 w269]
              tunnel: [w253 w262] -> w237
              tunnel: w236 -> [w253 w268]
              tunnel: [w252 w261] -> w235
              tunnel: w234 -> [w252 w267]
              tunnel: w233 -> [w251 w259]
              frame False {
              }
              frame True {
                n108 = To Long Integer(number=w274) -> (32bit integer=w260:i32)
                n109 = for {
                  N: w260 -> [_]
                  shift-right: [w304] -> w273
                  shift-left: w275 -> [w303]
                  shift-right: [w297] -> w266
                  shift-left: w272 -> [w298]
                  shift-right: [w296] -> w265
                  shift-left: w271 -> [w295]
                  shift-right: [w289] -> w264
                  shift-left: w270 -> [w290]
                  shift-right: [w288] -> w263
                  shift-left: w269 -> [w287]
                  shift-right: [w281] -> w262
                  shift-left: w268 -> [w282]
                  shift-right: [w280] -> w261
                  shift-left: w267 -> [w279]
                  w276 = 1 ("n")
                  n110 = Rotate 1D Array(1:w298, 2:w276) -> (0:w299:dbl[])
                  n111 = Rotate 1D Array(1:w303, 2:w276) -> (0:w302:dbl[])
                  n112 = Rotate 1D Array(1:w290, 2:w276) -> (0:w291:dbl[])
                  n113 = Rotate 1D Array(1:w287, 2:w276) -> (0:w286:dbl[])
                  n114 = Rotate 1D Array(1:w295, 2:w276) -> (0:w294:dbl[])
                  n115 = Rotate 1D Array(1:w282, 2:w276) -> (0:w283:T4)
                  n116 = Rotate 1D Array(1:w279, 2:w276) -> (0:w278:T4)
                  n117 = Index Array(array=w299) -> (element=w300:dbl)  [unwired: 1 in]
                  n118 = Index Array(array=w302) -> (element=w301:dbl)  [unwired: 1 in]
                  n119 = Index Array(array=w291) -> (element=w292:dbl)  [unwired: 1 in]
                  n120 = Index Array(array=w286) -> (element=w285:dbl)  [unwired: 1 in]
                  n121 = Index Array(array=w294) -> (element=w293:dbl)  [unwired: 1 in]
                  n122 = Index Array(array=w283) -> (element=w284:T3)  [unwired: 1 in]
                  n123 = Index Array(array=w278) -> (element=w277:T3)  [unwired: 1 in]
                  n124 = Insert Into Array(array=w298, new element=w300) -> (w297:dbl[])  [unwired: 1 in]
                  n125 = Insert Into Array(array=w303, new element=w301) -> (w304:dbl[])  [unwired: 1 in]
                  n126 = Insert Into Array(array=w290, new element=w292) -> (w289:dbl[])  [unwired: 1 in]
                  n127 = Insert Into Array(array=w287, new element=w285) -> (w288:dbl[])  [unwired: 1 in]
                  n128 = Insert Into Array(array=w295, new element=w293) -> (w296:dbl[])  [unwired: 1 in]
                  n129 = Insert Into Array(array=w282, new element=w284) -> (w281:T4)  [unwired: 1 in]
                  n130 = Insert Into Array(array=w279, new element=w277) -> (w280:T4)  [unwired: 1 in]
                }
              }
            }
            n131 = in-place-cluster #3("Record Length"=w248, "CHC"=w247, "u m/s"=w245, "v m/s"=w243, "time s"=w241, "Vel mag m/s"=w239, "Turb Stats Error"=w237, "Turb Stats"=w235) -> (w229:T2)
          }
        }
      }
      frame "Create Files" {
        n132 = Index Array(array=w318) -> (element=w332:T2)  [unwired: 1 in]
        n133 = Equal?(x=w313, y=1) -> (x = y?=w307:bool)
        n134 = Build Path(base path=w334, name or relative path=w335) -> (appended path=w310:path)
        n135 = call "Get Cluster Element Names.vi"("Cluster"=w332) -> ("Element Names"=w331:string[])  [unwired: 9 in, 1 out]
        n136 = Unbundle By Name(w332) -> ("Turb Stats"=w322:T4)
        n137 = call <vilib>:"Check if File or Folder Exists.vi"("path"=w310) -> ("file or folder exists?"=w308:bool, "dup path"=w309:path)  [unwired: 8 in, 1 out]
        n138 = And(x=w307, y=w308) -> (x .and. y?=w306:bool)
        n139 = case shown="True" w306 {
          tunnel: [w339 w341] -> w305
          tunnel: w309 -> [w339 w340]
          frame False {
          }
          frame True {
            n140 = Delete(path (use dialog)=w340) -> (deleted path=w341:path)  [unwired: 4 in, 2 out]
          }
        }
        n141 = Delete From Array(array=w331, length=3, index=6) -> (deleted portion=w317:string[], array with subset deleted=w327:string[])
        n142 = Index Array(array=w322) -> (element=w321:T3)  [unwired: 1 in]
        n143 = call "Get Cluster Element Names.vi"("Cluster"=w321) -> ("Element Names"=w328:string[])  [unwired: 9 in, 1 out]
        n144 = Delete From Array(array=w317, length=1, index=0) -> (array with subset deleted=w316:string[])  [unwired: 1 out]
        n145 = for {
          tunnel: w316 -> [w344] mode=indexing
          tunnel: w328 -> [w343]
          tunnel: [w342] -> w326 mode=indexing
          n146 = for {
            tunnel: w344 -> [w348]
            tunnel: w343 -> [w346] mode=indexing
            tunnel: [w345] -> w342 mode=indexing
            n147 = Concatenate Strings(w348, "_" ("string"), w346) -> (w345:string)
          }
        }
        n148 = Index Array(array=w326) -> (element #1=w325:string[], element #2=w324:string[])  [unwired: 4 in]
        n149 = Build Path(base path=w305, name or relative path="ENSI_all.case") -> (appended path=→"ALL filepath":path)
        n150 = Build Array (concatenate)(w327, w325, w324) -> (w323:string[])
        n151 = for {
          tunnel: w323 -> [w351] mode=indexing
          tunnel: [w353] -> w320 mode=indexing
          w357 = "_" ("Replace with")
          n152 = call <vilib>:"Trim Whitespace.vi"("string"=w351) -> ("trimmed string"=w349:string)  [unwired: 1 in]
          n153 = call "Replace_Character.vi"("Replace with"="_", "Input String"=w349, "Search For"=" ") -> ("Output string"=w352:string)  [unwired: 1 out]
          n154 = call "Replace_Character.vi"("Replace with"=w357, "Input String"=w352, "Search For"="(") -> ("Output string"=w359:string)  [unwired: 1 out]
          n155 = call "Replace_Character.vi"("Replace with"=w357, "Input String"=w359, "Search For"=")") -> ("Output string"=w356:string)  [unwired: 1 out]
          n156 = call "Replace_Character.vi"("Replace with"="", "Input String"=w356, "Search For"="/") -> ("Output string"=w353:string)  [unwired: 1 out]
        }
        "Variable Names" <- w320
        n157 = local read "Max Record Length"() -> (w319:i32)
        n158 = for {
          N: w319 -> [_]
          tunnel: w305 -> [w379]
          tunnel: w320 -> [w378]
          tunnel: [w377] -> w338 mode=indexing
          i -> [w373]
          n159 = Number To Decimal String(number=w373, width (-)=i16 4) -> (decimal integer string=w371:string)
          n160 = call "Whitespace_to_Zeros.vi"("Input String"=w371) -> ("Output String"=w367:string)  [unwired: 6 in]
          n161 = Concatenate Strings("ENSI_" ("name or relative path"), w367) -> (w363:string)
          n162 = Concatenate Strings(w363, ".var" ("name or relative path")) -> (w362:string)
          n163 = for {
            tunnel: w379 -> [w386]
            tunnel: [w381] -> w374 mode=indexing
            tunnel: w378 -> [_] mode=indexing
            tunnel: w362 -> [w380]
            i -> [w385]
            n164 = Increment(x=w385) -> (x+1=w384:i32)
            n165 = Number To Decimal String(number=w384) -> (decimal integer string=w383:string)  [unwired: 1 in]
            n166 = Concatenate Strings(w380, w383) -> (w382:string)
            n167 = Build Path(base path=w386, name or relative path=w382) -> (appended path=w381:path)
          }
          n168 = Concatenate Strings(w363, ".case" ("name or relative path")) -> (w370:string)
          n169 = Concatenate Strings(w363, ".geo" ("name or relative path")) -> (w366:string)
          n170 = Build Path(base path=w379, name or relative path=w370) -> (appended path=w375:path)
          n171 = Build Path(base path=w379, name or relative path=w366) -> (appended path=w376:path)
          n172 = Build Array (concatenate)(w375, w376, w374) -> (w377:path[])
        }
        "File Paths" <- w338
      }
      frame "Setup Files" {
        n173 = local read "File Paths"() -> (w390:path[][])
        n174 = for {
          tunnel: w390 -> [w395] mode=indexing
          i -> [w392]
          n175 = Number To Decimal String(number=w392, width (-)=i16 4) -> (decimal integer string=w393:string)
          n176 = call "Whitespace_to_Zeros.vi"("Input String"=w393) -> ("Output String"=w391:string)  [unwired: 6 in]
          n177 = for {
            tunnel: w395 -> [w398] mode=indexing
            tunnel: w391 -> [w396]
            i -> [w397]
            n178 = case shown="1" w397 {
              tunnel: w398 -> [w409 w434 w453]
              tunnel: w397 -> [_ _ w448]
              tunnel: w396 -> [w399 _ _]
              frame 0 {
                n179 = local read "Variable Names"() -> (w413:string[])
                n180 = for {
                  tunnel: w413 -> [w425] mode=indexing
                  tunnel: [w423] -> w408 mode=indexing
                  tunnel: w399 -> [w420]
                  i -> [w427]
                  n181 = Increment(x=w427) -> (x+1=w428:i32)
                  n182 = Concatenate Strings(" ENSI_.var", w420, ".var") -> (w422:string)
                  n183 = Number To Decimal String(number=w428) -> (decimal integer string=w426:string)  [unwired: 1 in]
                  n184 = Concatenate Strings(w422, w426) -> (w424:string)
                  n185 = Concatenate Strings("scalar per node: ", w425, w424) -> (w423:string)
                }
                n186 = Concatenate Strings("model: ENSI_", w399, ".geo") -> (w401:string)
                n187 = Build Array (concatenate)("FORMAT", "type: ensight gold", "GEOMETRY", w401, "VARIABLE", w408) -> (w407:string[])
                n188 = for {
                  tunnel: w407 -> [w418] mode=indexing
                  shift-right: [w416] -> w411
                  shift-left: "" -> [w414]
                  n189 = Concatenate Strings(w418, "\r\n") -> (w415:string)
                  n190 = Concatenate Strings(w414, w415) -> (w416:string)
                }
                n191 = call "Write_File_Simple.vi"("append to file? (new file:F)"=FALSE, "character string"=w411, "file path"=w409) -> ()  [unwired: 2 out]
              }
              frame 1 {
                n192 = local read "# total vectors"() -> (w432:i32)
                n193 = Number To Decimal String(number=w432) -> (decimal integer string=w431:string)  [unwired: 1 in]
                n194 = Build Array (concatenate)(string[] ["EnSight Model Geometry File", "EnSight 9.2 ", "node id assign", "element id assign", "part", "         1", "Point field", "coordinates"], w431) -> (w430:string[])
                n195 = for {
                  tunnel: w430 -> [w442] mode=indexing
                  shift-right: [w440] -> w436
                  shift-left: "" -> [w438]
                  n196 = Concatenate Strings(w442, "\r\n") -> (w439:string)
                  n197 = Concatenate Strings(w438, w439) -> (w440:string)
                }
                n198 = call "Write_File_Simple.vi"("append to file? (new file:F)"=FALSE, "character string"=w436, "file path"=w434) -> ()  [unwired: 2 out]
              }
              frame 2, Default {
                n199 = local read "Variable Names"() -> (w449:string[])
                n200 = Subtract(x=w448, y=2) -> (x-y=w446:i32)
                n201 = Index Array(array=w449, index=w446) -> (element=w445:string)
                n202 = Build Array (concatenate)(w445, string[] ["part", "         1", "coordinates"]) -> (w443:string[])
                n203 = for {
                  tunnel: w443 -> [w458] mode=indexing
                  shift-right: [w456] -> w451
                  shift-left: "" -> [w454]
                  n204 = Concatenate Strings(w458, "\r\n") -> (w455:string)
                  n205 = Concatenate Strings(w454, w455) -> (w456:string)
                }
                n206 = call "Write_File_Simple.vi"("append to file? (new file:F)"=FALSE, "character string"=w451, "file path"=w453) -> ()  [unwired: 2 out]
              }
            }
          }
        }
      }
      frame "Collect Data" {
        n207 = local read "Max Record Length"() -> (w464:i32)
        n208 = local read "ALL filepath"() -> (w465:path)
        n209 = Number To Decimal String(number=w464) -> (decimal integer string=w468:string)  [unwired: 1 in]
        n210 = for {
          tunnel: w463 -> [w482] mode=indexing
          tunnel: [w472] -> w462 mode=indexing
          tunnel: [w471] -> w460 mode=indexing
          i -> [w481]
          n211 = Unbundle By Name(w482) -> ("Record Length"=w480:dbl, "CHC"=w479:dbl[], "u m/s"=w478:dbl[], "v m/s"=w477:dbl[], "time s"=w476:dbl[], "Vel mag m/s"=w475:dbl[], "Turb Stats"=w474:T4, "Turb Stats Error"=w473:T4, "XYZ Position"=w471:dbl[])
          n212 = for {
            tunnel: w480 -> [w493]
            tunnel: w479 -> [w492] mode=indexing
            tunnel: w478 -> [w491] mode=indexing
            tunnel: w477 -> [w490] mode=indexing
            tunnel: w476 -> [w489] mode=indexing
            tunnel: w475 -> [w488] mode=indexing
            tunnel: w474 -> [w487] mode=indexing
            tunnel: w473 -> [w485] mode=indexing
            tunnel: [w483] -> w472 mode=indexing
            n213 = Cluster To Array(cluster=w487) -> (array=w486:dbl[])
            n214 = Cluster To Array(cluster=w485) -> (array=w484:dbl[])
            n215 = Build Array (concatenate)(w493, w492, w491, w490, w489, w488, w486, w484) -> (w483:dbl[])
          }
          "Collect data" <- w481
        }
        "Data Array" <- w462
        n216 = call <vilib>:"Check if File or Folder Exists.vi"("path"=w465) -> ("file or folder exists?"=w466:bool, "dup path"=w467:path)  [unwired: 8 in, 1 out]
        n217 = case shown="False" w466 {
          tunnel: w467 -> [w518 _]
          tunnel: w468 -> [w503 _]
          tunnel: w464 -> [w496 _]
          frame False {
            n218 = local read "Tmax"() -> (w494:dbl)
            n219 = local read "Variable Names"() -> (w510:string[])
            n220 = call-poly <vilib>:"Ramp Pattern.vi"("end"=w494, "samples"=w496) -> ("Ramp Pattern"=w495:dbl[])  [unwired: 8 in, 1 out]
            n221 = for {
              tunnel: w510 -> [w527] mode=indexing
              tunnel: [w525] -> w509 mode=indexing
              i -> [w529]
              n222 = Increment(x=w529) -> (x+1=w530:i32)
              n223 = Number To Decimal String(number=w530) -> (decimal integer string=w528:string)  [unwired: 1 in]
              n224 = Concatenate Strings(" ENSI_***.var", w528) -> (w526:string)
              n225 = Concatenate Strings("scalar per node: ", w527, w526) -> (w525:string)
            }
            n226 = Concatenate Strings("number of steps: ", w503) -> (w501:string)
            n227 = Number To Fractional String(number=w495, precision (6)=i16 1) -> (F-format string=w497:string[])  [unwired: 2 in]
            n228 = Build Array (concatenate)("FORMAT", "type: ensight gold", "GEOMETRY", "model: ENSI_***.geo", "VARIABLE", w509, "TIME", "time set: 1", w501, "filename start number: 000", "filename increment: 001", "time values:", w497) -> (w506:string[])
            n229 = for {
              tunnel: w506 -> [w523] mode=indexing
              shift-right: [w521] -> w507
              shift-left: "" -> [w519]
              n230 = Concatenate Strings(w523, "\r\n") -> (w520:string)
              n231 = Concatenate Strings(w519, w520) -> (w521:string)
            }
            n232 = call "Write_File_Simple.vi"("append to file? (new file:F)"=FALSE, "character string"=w507, "file path"=w518) -> ()  [unwired: 2 out]
          }
          frame True {
          }
        }
        n233 = Transpose 2D Array(2D array=w460) -> (transposed array=w459:dbl[][])
        "Position Array" <- w459
        n234 = Array Size(array=w459) -> (size(s)=→"size(s)":i32[])
      }
      frame "Save Data" {
        n235 = local read "File Paths"() -> (w534:path[][])
        n236 = local read "Position Array"() -> (w532:dbl[][])
        n237 = local read "Data Array"() -> (w533:dbl[][][])
        n238 = for {
          tunnel: w534 -> [w541] mode=indexing
          tunnel: w533 -> [w540]
          tunnel: w532 -> [w538]
          i -> [w539]
          # "Loop Time"
          n239 = for {
            tunnel: w541 -> [w546] mode=indexing
            tunnel: w540 -> [w545]
            tunnel: w539 -> [w544]
            tunnel: w538 -> [w542]
            i -> [w543]
            # "Loop Variable"
            n240 = case shown="1" w543 {
              tunnel: w546 -> [_ w552 w563]
              tunnel: w543 -> [_ _ w572]
              tunnel: w545 -> [_ _ w569]
              tunnel: w544 -> [_ _ w567]
              tunnel: w542 -> [_ w551 _]
              frame 0 {
              }
              frame 1 {
                n241 = Index Array(array=w551) -> (element #1=w550:dbl[], element #2=w549:dbl[], element #3=w548:dbl[])  [unwired: 6 in]
                n242 = Build Array (concatenate)(w550, w549, w548) -> (w547:dbl[])
                n243 = for {
                  tunnel: w547 -> [w556] mode=indexing
                  shift-right: [w562] -> w553
                  shift-left: "" -> [w561]
                  w557 = T5 4 items=["no dialog", "OK message", "continue or stop message", "OK message + warnings", "continue/stop + warnings"] ("type of dialog (OK msg:1)")
                  (unwired) "%0.5e" ("format string")
                  n244 = call "Ensight_Format_Check.vi"("Input Number"=w556) -> ("error"=w559:errorcluster, "Output string"=w560:string)  [unwired: 8 in, 1 out]
                  n245 = Concatenate Strings(w561, w560) -> (w562:string)
                  n246 = call <vilib>:"Simple Error Handler.vi"("error source (\" \")"="GEOM" ("error source (\" \")"), "type of dialog (OK msg:1)"=w557, "error in (no error)"=w559) -> ()  [unwired: 2 in, 5 out]
                }
                n247 = call "Write_File_Simple.vi"("append to file? (new file:F)"=TRUE, "character string"=w553, "file path"=w552) -> ()  [unwired: 2 out]
              }
              frame 2, Default {
                n248 = Subtract(x=w572, y=2) -> (x-y=w568:i32)
                n249 = Index Array(array=w569, index (dim 1)=w567, index (dim 2)=w568) -> (element=w566:dbl[])  [unwired: 1 in]
                n250 = for {
                  tunnel: w566 -> [w573] mode=indexing
                  shift-right: [w582] -> w564
                  shift-left: "" -> [w581]
                  tunnel: w563 -> [w578]
                  w574 = T5 4 items=["no dialog", "OK message", "continue or stop message", "OK message + warnings", "continue/stop + warnings"] ("type of dialog (OK msg:1)")
                  n251 = Path To String(path=w578) -> (string=w577:string)
                  n252 = call "Ensight_Format_Check.vi"("Input Number"=w573) -> ("error"=w579:errorcluster, "Output string"=w580:string)  [unwired: 8 in, 1 out]
                  n253 = Concatenate Strings("VAR file: " ("error source (\" \")"), w577) -> (w575:string)
                  n254 = call <vilib>:"Simple Error Handler.vi"("error source (\" \")"=w575, "type of dialog (OK msg:1)"=w574, "error in (no error)"=w579) -> ()  [unwired: 2 in, 5 out]
                  n255 = Concatenate Strings(w581, w580) -> (w582:string)
                }
                n256 = call "Write_File_Simple.vi"("append to file? (new file:F)"=TRUE, "character string"=w564, "file path"=w563) -> ()  [unwired: 2 out]
              }
            }
            "Variable Loop" <- w543
          }
          "Time Loop" <- w539
        }
      }
    }
  }
